vi "Anna_linescan2.0.vi"() -> ()   [LabVIEW 2009]
panel:
  in  "stop batch":bool
  in  "first scan?":bool
  in  "Batch Analyze":bool
  in  "Case Constant\n(See Context Help)":bool
  in  "Router":u32
  in  "save image to txt file":bool
  in  "threshold":cluster{"max":u32, "min":u32}={"max"=100, "min"=20}
  in  "Header Path Ring":u16(ring)
  out "spots":i16
  in  "notes":string="file: 5\r\n13.07.2011 11:31:22\r\n\r\n83 spot(s) found\r\nclose filter:  TRUE\r\nconnectivity 4/8: TRUE\r\nthreshold (min):  20\r\nthreshold (max):  200\r\nselection values:\r\n\r\nNo spots stored.\r\n83 spot(s) found\r\nclose filter:  TRUE\r\nconnectivity 4/8: TRUE\r\nthreshold (min):  20\r\nthreshold (max):  200\r\nselection values:\r\n\r\nNo spots stored.\r\n\r\n\r\nfile: 5\r\n15.07.2011 16:28:43\r\n"
  in  "new image":bool
  in  "exit":bool
  out "does a coinc image exist?":bool
  in  "coincidence spot":bool
  in  "coincidence\nimage":bool
  out "LOADED HDR":bool=TRUE
  out "Image LOADED":bool=TRUE
  in  "settings":bool
  in  "Load Image":bool
  in  "F2-Image":bool
  in  "Lifetime pick":bool
  in  "Export":bool
  in  "TAC Window":bool
  in  "Spotfinder":bool
  in  "View FIFO Settings":bool
  in  "View Image Settings":bool
  in  "Load":bool
  out "total":i32=502376
  out "gap":i32
  out "invalid":i32=69
  in  "plane":u32
  in  "router":u8(ring) items=["sum", "0", "1", "2", "3", "4", "5"]
  in  "RGB or false color?":bool
  in  "16bit":bool
  out "already x spots":i16
  out "Int duplex?":bool
  out "16btimage?":bool
  out "Ampel":cluster{"RED":bool, "YELLOW":bool, "GREEN":bool}={"RED"=FALSE, "YELLOW"=FALSE, "GREEN"=TRUE}
  out "TACwinLoaded?":bool=TRUE
  out "Boolean":bool=TRUE
  in  "Image Path":path=path "C:/Users/Phil/Desktop/11_07_08 Guillermo correlations/silver 40 nm/5/5.hdr"
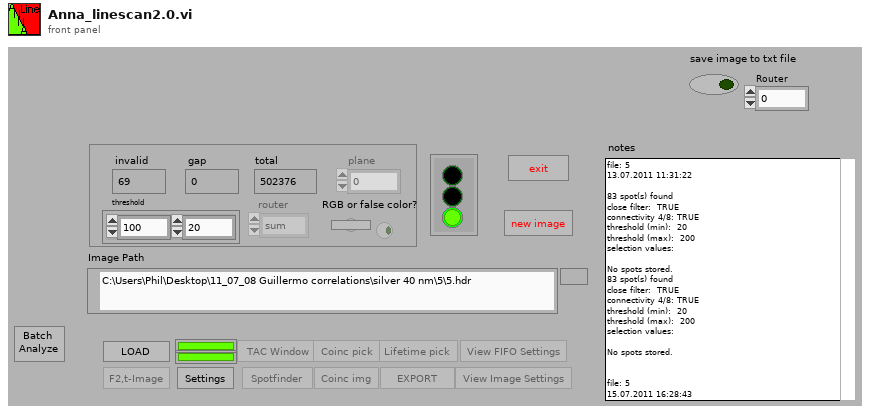
[diagram p1: front panel]
types:
  T1 = enum16{"Display", "change", "get", "save", "create text", "load", "Get Refnum"}
  T2 = enum16{"Get", "Set", "Change", "ini", "clear", "draw", "draw false"}
  T3 = enum16{"Ini", "Get", "Set", "Refresh", "dump", "move", "name"}
  T4 = enum16{"Ini", "Dump", "Colorpal", "Input", "Get"}
  T5 = enum16{"Display", "change", "Get", "Set", "Set Ken"}
  T6 = enum8{"Enabled", "Disabled", "Disabled and Grayed Out"}
  T7 = enum16{"Ini", "Get", "Set", "Draw", "Colorpal", "Dump", "Zoom"}
  T8 = cluster{"router":u8[], "macro times":dbl[], "micro times":u16[], "invalid":dbl[], "gap":dbl[]}
  T9 = typedef "Settings.ctl" = cluster{"threshold":cluster{"max":u32, "min":u32}, "RGB or false color":bool, "16bit":bool, "log/lin axis":u16, "spotsize button":bool, "Pixelsize":u16, "autoscale x":bool, "autoscale y":bool, "correlation":bool, "ADC-Resolution":i32, "F2-lifetime":cluster{"display tau":bool, "display F2":bool, "Palette Number lifetime":enum32{"Gray", "Binary", "Gradient", "Rainbow", "Temperature"}, "Palette Number F2":enum32{"Gray", "Binary", "Gradient", "Rainbow", "Temperature"}, "max tau-Value":dbl, "min tau-Value":dbl, "max F2-Value":dbl, "min F2-Value":dbl}, "TAC-Window 1":u16, "TAC-Window 2":u16, "false color palette":cluster{"1":u32, "2":u32, "3":u32, "4":u32, "5":u32, "6":u32, "7":u32, "8":u32, "8 2":u32, "8 3":u32, "8 4":u32, "8 5":u32}, "rebinning":dbl}
  T10 = enum32{"existing file", "new file", "new or existing file", "existing dir", "new dir", "new or existing dir", "existing file (use LLBs)", "new file (use LLBs)", "new or existing file (use LLBs)", "new or existing file or directory (use LLBs)"}
  T11 = typedef "ImageSettings.ctt" = cluster{"Start Position (µm)":cluster{"x":dbl, "y":dbl, "z":dbl}, "End Position (µm)":cluster{"x":dbl, "y":dbl, "z":dbl}, "Image Resolution (nm/pixel)":cluster{"x":dbl, "y":dbl, "z":dbl}, "Image Size (µm)":cluster{"x":dbl, "y":dbl, "z":dbl}, "Image Size (pixel)":cluster{"x":u32, "y":u32, "z":u32}, "Time Resolution\n(ms/pixel)":dbl, "1st Axis":u16, "2nd Axis":u16, "Retrace":bool, "Estimated Time":string}
  T12 = typedef "FIFOSettings_BH.ctt" = cluster{"Measurement":cluster{"Binning (ms)":sgl, "External Trigger Condition":u16, "Stop Condition:":u16, "Stop Count":dbl, "Buffer Size (Photons)":u16, "No of Channels":u16, "Ext Latch Delay":i16}, "ADC":cluster{"Module":u16, "ADC Resolution":i32, "Dither Range":i16, "Count Increment":i16, "Macro Time Clock":i16}, "SYNC":cluster{"SYNC ZC Level (mV)":sgl, "SYNC Freq Divider":i16, "SYNC Holdoff (ns)":sgl, "SYNC Threshold (mV)":sgl}, "TAC":cluster{"TAC Range (ns)":sgl, "TAC Gain":i16, "TAC Offset (%)":sgl, "TAC Limit Low (%)":sgl, "TAC Limit High (%)":sgl}, "CFD":cluster{"CFD Limit Low (mV)":sgl, "CFD Limit High (mV)":sgl, "CFD ZC Level (mV)":sgl, "CFD Holdoff (ns)":sgl}}
  T13 = typedef "spotproperties.ctl" = cluster{"draw?":bool, "plane":u32, "Coordinates":i32[], "TACWindow":cluster{"TACWindow1":i32, "TACWindow2":i32}, "Lifetime[ns]":ext[], "tauerror":dbl[], "F2-Value overall":dbl, "overall intensity":u32[], "F2-Value TAC":dbl, "TAC intensity":u32[], "Decay":u32[][]}
  T14 = enum16{"open", "replace", "create", "open or create", "replace or create", "replace or create with confirmation"}
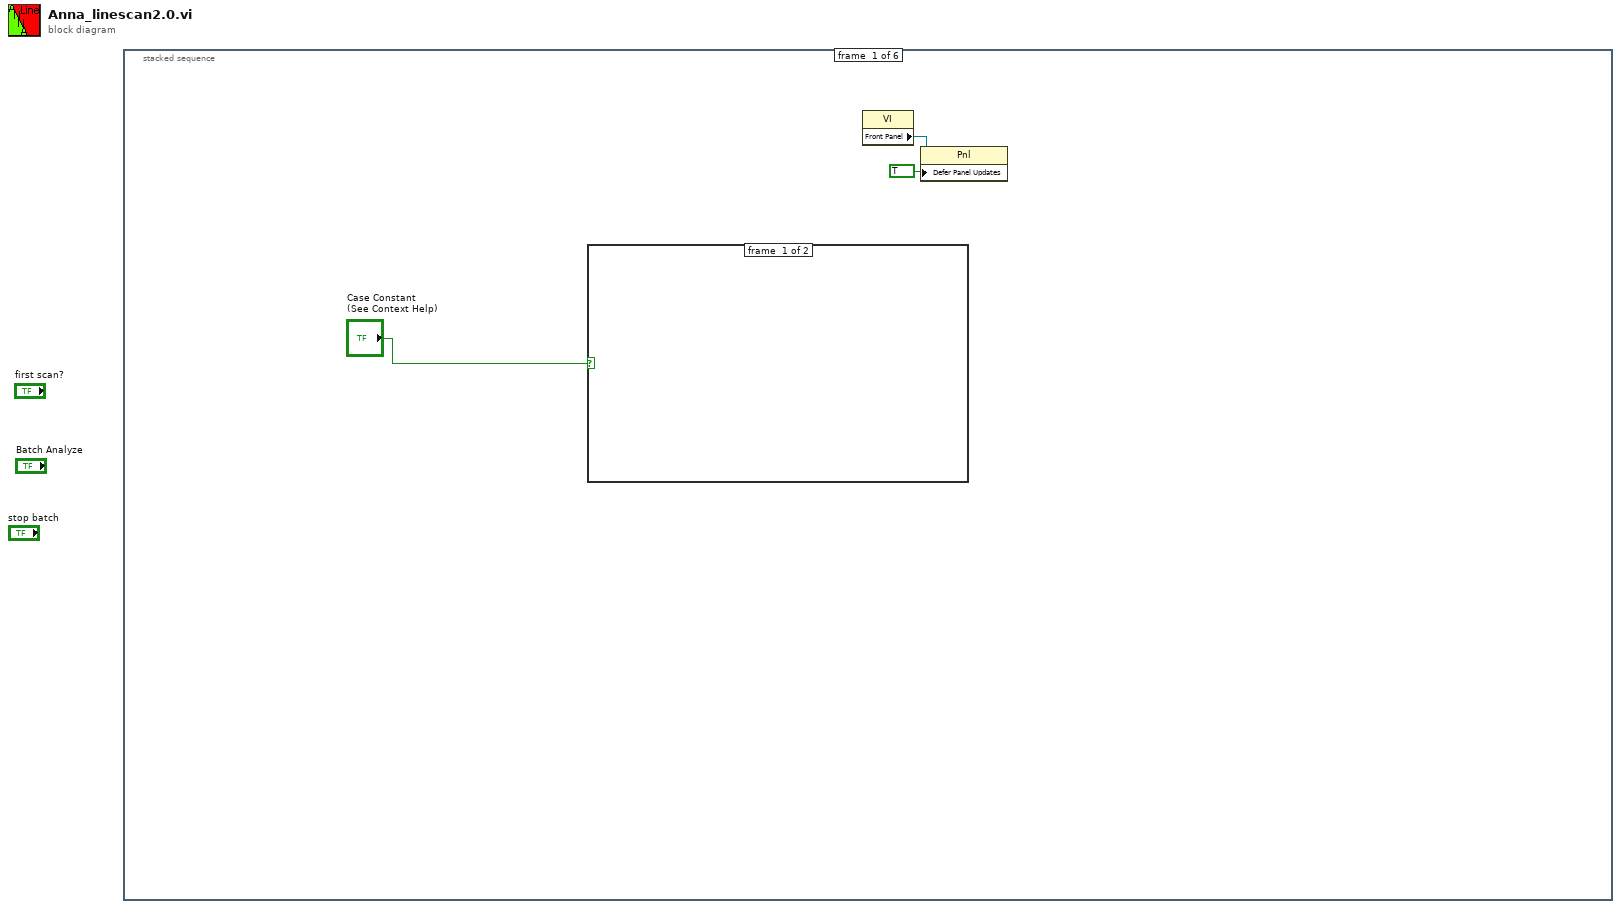
[diagram p0: block diagram]
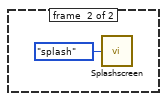
[diagram p2: hidden frame]
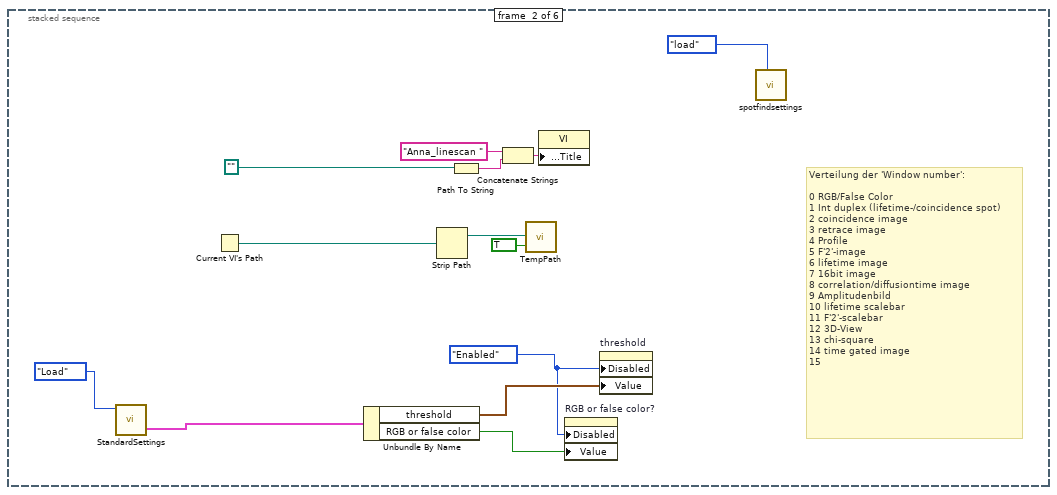
[diagram p3: hidden frame]
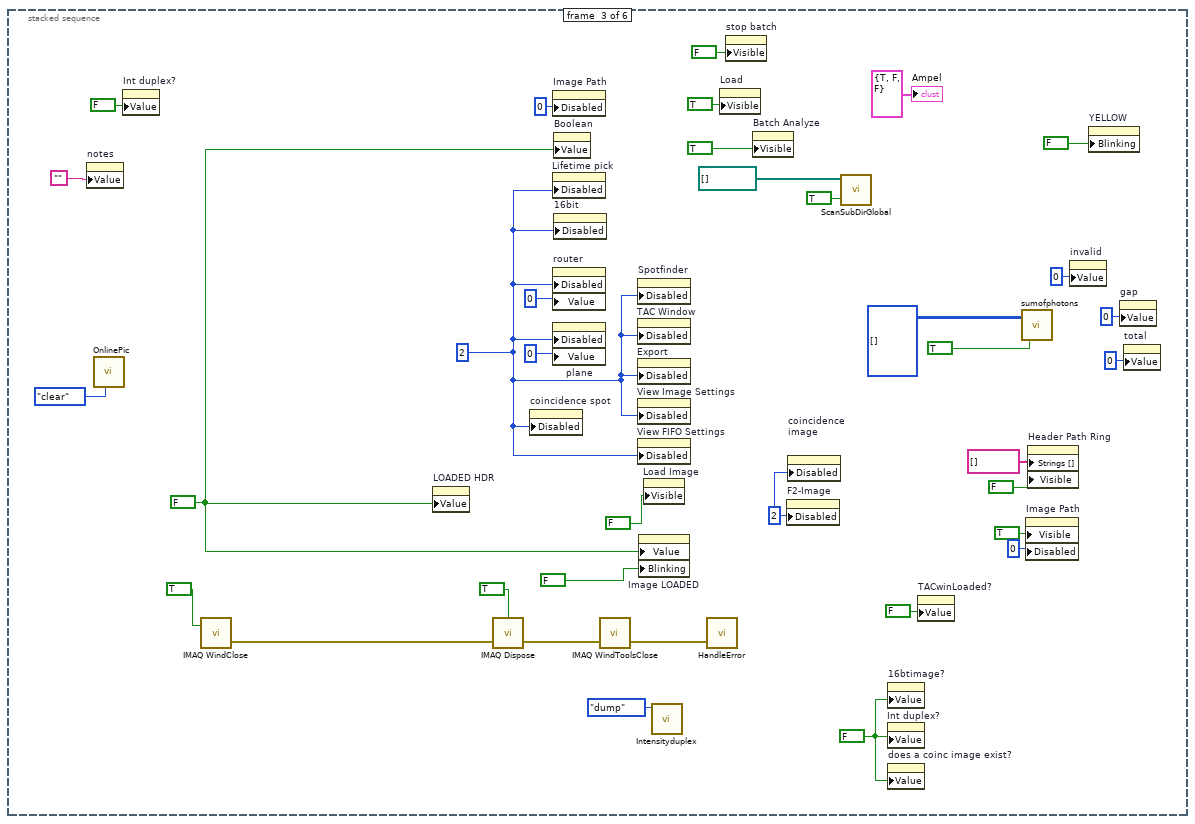
[diagram p4: hidden frame]
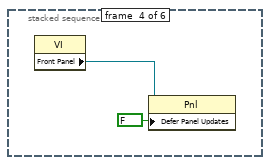
[diagram p5: hidden frame]
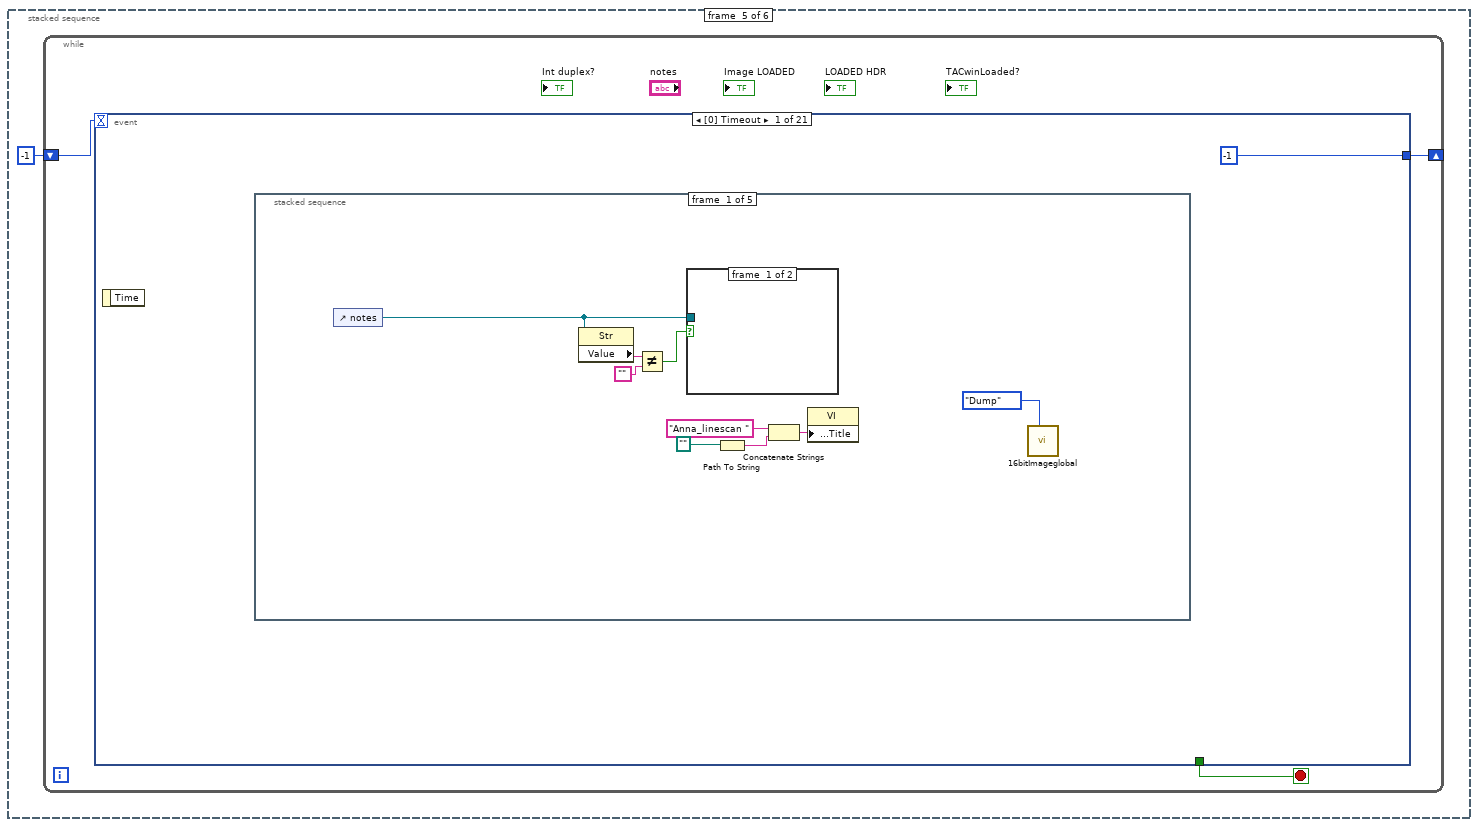
[diagram p6: hidden frame]
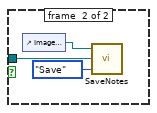
[diagram p7: hidden frame]
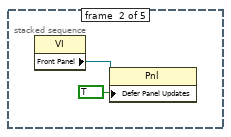
[diagram p8: hidden frame]
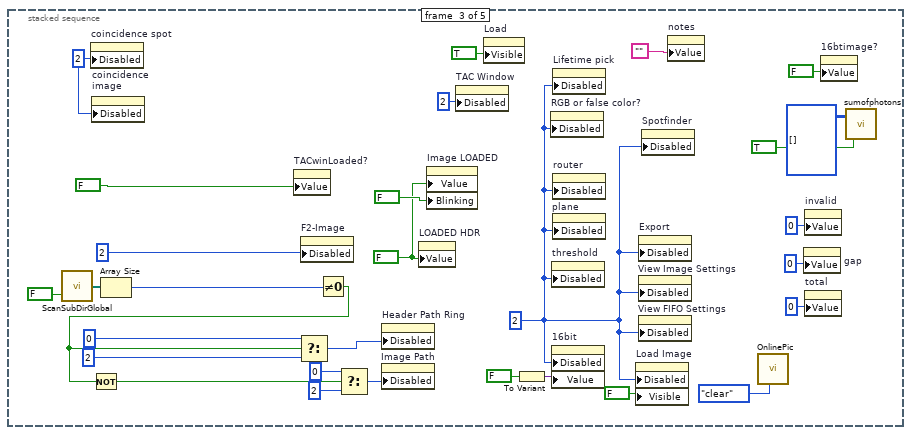
[diagram p9: hidden frame]
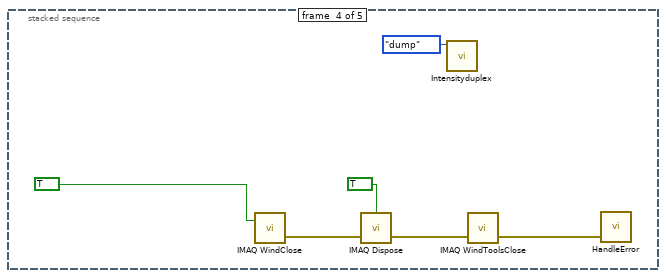
[diagram p10: hidden frame]
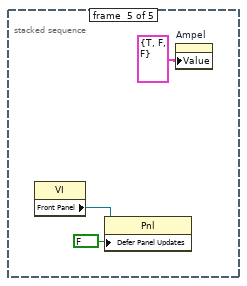
[diagram p11: hidden frame]
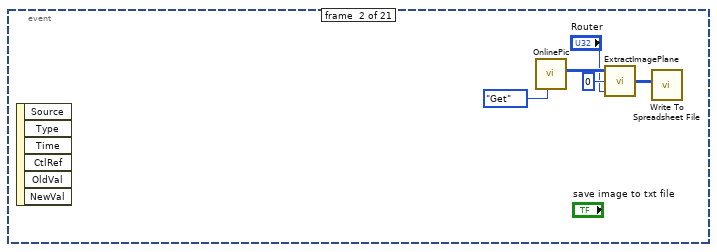
[diagram p12: hidden frame]
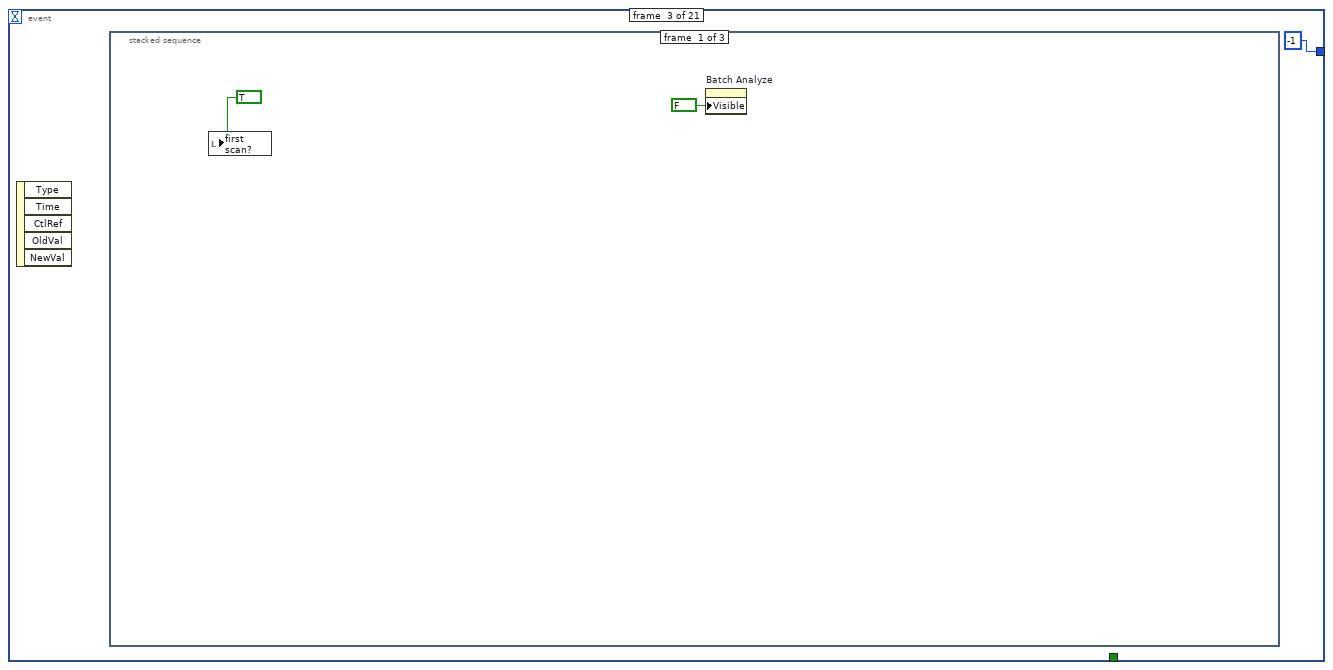
[diagram p13: hidden frame]
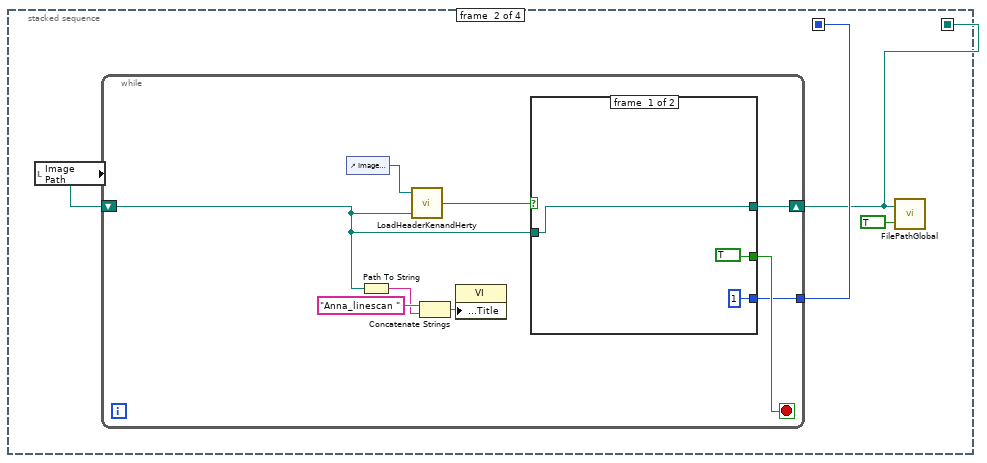
[diagram p15: hidden frame]
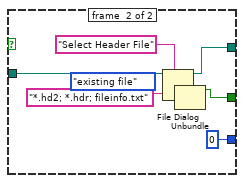
[diagram p16: hidden frame]
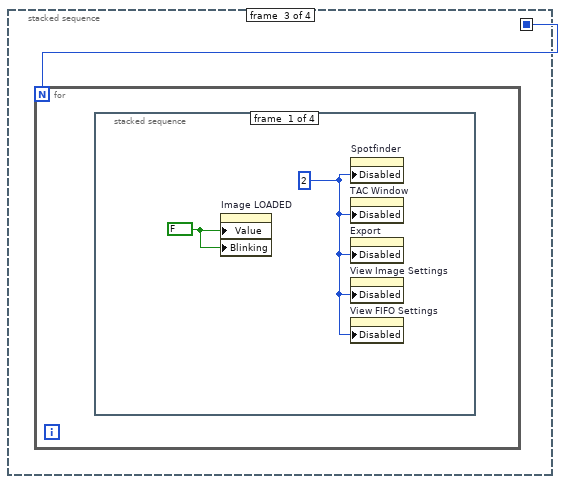
[diagram p17: hidden frame]
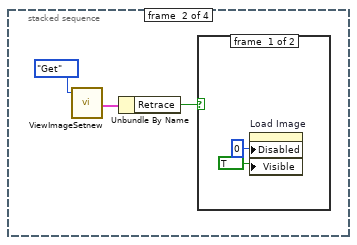
[diagram p18: hidden frame]
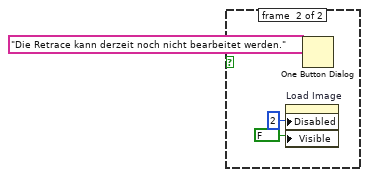
[diagram p19: hidden frame]
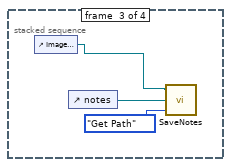
[diagram p20: hidden frame]
diagram:
  n1 = stacked-sequence {
    frame #0 {
      n2 = case shown="False" "Case Constant\n(See Context Help)" {
        frame #0 {
        }
        frame #1 {
          n3 = call "Splashscreen.vi"("Mode"=enum16{"splash", "dialog"}."splash") -> ()  [unwired: 1 in]
        }
      }
      n4 = property class="VI"() -> ("Front Panel"=w2:refnum<vi>)  [unwired: 2 in, 2 out]
      n5 = property class="Pnl"(reference=w2, "Defer Panel Updates"=TRUE) -> ()  [unwired: 1 in, 2 out]
    }
    frame #1 {
      w5 = T6."Enabled" ("Disabled")
      # "Verteilung der 'Window number':\n\n0 RGB/False Color\n1 Int duplex (lifetime-/coincidence spot)\n2 coincidence image\n3 retrace image\n4 Profile\n5 F'2'-image\n6 lifetime image\n7 16bit image\n8 correlation/diffusiontime image\n9 Amplitudenbild\n10 lifetime scalebar\n11 F'2'-scalebar\n12 3D-View\n13 chi-square\n14 time gated image\n15"
      n6 = call "StandardSettings.vi"("Enum"=enum16{"Load", "get", "Save", "set"}."Load") -> ("StandardSettings"=w7:T9)  [unwired: 4 in]
      n7 = Current VI's Path() -> (path=w17:path)
      n8 = Unbundle By Name(w7) -> ("threshold"=w6:cluster{"max":u32, "min":u32}, "RGB or false color"=w8:bool)
      n9 = Strip Path(path=w17) -> (stripped path=w16:path)  [unwired: 1 out]
      n10 = Path To String(path=path "") -> (string=w12:string)
      n11 = Concatenate Strings("Anna_linescan " ("string"), w12) -> (w14:string)
      n12 = call "TempPath.vi"("change"=TRUE, "stripped path"=w16) -> ()  [unwired: 1 in, 1 out]
      n13 = property class="VI"("Front Panel Window:Title"=w14) -> ()  [unwired: 2 in, 2 out]
      n14 = property on="RGB or false color?" class="Boolean (strict)"("Disabled"=w5, "Value"=w8) -> ()  [unwired: 2 in, 2 out]
      n15 = property on="threshold" class="Clust (strict)"("Disabled"=w5, "Value"=w6) -> ()  [unwired: 2 in, 2 out]
      n16 = call "spotfindsettings.vi"("Enum"=T1."load") -> ()  [unwired: 8 in, 3 out]
    }
    frame #2 {
      w33 = FALSE
      w32 = u8 2 ("Disabled")
      w44 = FALSE ("Boolean")
      w22 = u8 2 ("Disabled")
      n17 = property on="notes" class="String"("Value"="") -> ()  [unwired: 2 in, 2 out]
      n18 = call "OnlinePic.vi"("action"=T2."clear" ("Enum")) -> ()  [unwired: 6 in, 5 out]
      n19 = property on="Int duplex?" class="Boolean (strict)"("Value"=FALSE ("Boolean 2")) -> ()  [unwired: 2 in, 2 out]
      n20 = call "IMAQ WindClose"("Close All Windows (False)"=TRUE ("Close All Windows (N)")) -> ("error out"=w49:errorcluster)  [unwired: 5 in]
      n21 = property on="LOADED HDR" class="Bool (strict)"("Value"=w44) -> ()  [unwired: 2 in, 2 out]
      n22 = call "IMAQ Dispose"("All Images? (No)"=TRUE, "error in (no error)"=w49) -> ("error out"=w50:errorcluster)  [unwired: 4 in]
      n23 = property on="coincidence spot" class="Boolean"("Disabled"=w22) -> ()  [unwired: 2 in, 2 out]
      n24 = property on="Image Path" class="Path"("Disabled"=u8 0) -> ()  [unwired: 2 in, 2 out]
      n25 = property on="Lifetime pick" class="Boolean"("Disabled"=w22) -> ()  [unwired: 2 in, 2 out]
      n26 = property on="router" class="Ring (strict)"("Disabled"=w22, "Value"=u8 0 ("router")) -> ()  [unwired: 2 in, 2 out]
      n27 = property on="plane" class="DigNum (strict)"("Disabled"=w22, "Value"=u32 0 ("plane")) -> ()  [unwired: 2 in, 2 out]
      n28 = property on="Boolean" class="Bool (strict)"("Value"=w44) -> ()  [unwired: 2 in, 2 out]
      n29 = property on="16bit" class="Boolean"("Disabled"=w22) -> ()  [unwired: 2 in, 2 out]
      n30 = call "IMAQ WindToolsClose"("error in (no error)"=w50) -> ("error out"=w48:errorcluster)  [unwired: 5 in]
      n31 = property on="Spotfinder" class="Boolean"("Disabled"=w22) -> ()  [unwired: 2 in, 2 out]
      n32 = property on="TAC Window" class="Boolean"("Disabled"=w22) -> ()  [unwired: 2 in, 2 out]
      n33 = property on="Export" class="Boolean"("Disabled"=w22) -> ()  [unwired: 2 in, 2 out]
      n34 = property on="View Image Settings" class="Boolean"("Disabled"=w22) -> ()  [unwired: 2 in, 2 out]
      n35 = property on="View FIFO Settings" class="Boolean"("Disabled"=w22) -> ()  [unwired: 2 in, 2 out]
      n36 = property on="Image LOADED" class="Boolean (strict)"("Value"=w44, "Blinking"=FALSE) -> ()  [unwired: 2 in, 2 out]
      n37 = property on="Load Image" class="Boolean"("Visible"=FALSE) -> ()  [unwired: 2 in, 2 out]
      n38 = call "Intensityduplex.vi"("Enum"=T3."dump") -> ()  [unwired: 4 in, 2 out]
      n39 = call "HandleError.vi"("error in (no error)"=w48) -> ()
      n40 = property on="Load" class="Bool"("Visible"=TRUE) -> ()  [unwired: 2 in, 2 out]
      n41 = property on="stop batch" class="Bool (strict)"("Visible"=FALSE) -> ()  [unwired: 2 in, 2 out]
      n42 = property on="Batch Analyze" class="Bool"("Visible"=TRUE) -> ()  [unwired: 2 in, 2 out]
      n43 = property on="F2-Image" class="Boolean"("Disabled"=w32) -> ()  [unwired: 2 in, 2 out]
      n44 = property on="coincidence\nimage" class="Bool"("Disabled"=w32) -> ()  [unwired: 2 in, 2 out]
      n45 = call "ScanSubDirGlobal.vi"("set"=TRUE, "Array 2"=path[] []) -> ()  [unwired: 1 out]
      n46 = property on="16btimage?" class="Boolean (strict)"("Value"=w33) -> ()  [unwired: 2 in, 2 out]
      n47 = property on="Int duplex?" class="Boolean (strict)"("Value"=w33) -> ()  [unwired: 2 in, 2 out]
      n48 = property on="does a coinc image exist?" class="Boolean (strict)"("Value"=w33) -> ()  [unwired: 2 in, 2 out]
      n49 = property on="TACwinLoaded?" class="Boolean (strict)"("Value"=FALSE ("TACwinLoaded?")) -> ()  [unwired: 2 in, 2 out]
      n50 = call "sumofphotons.vi"("s"=TRUE, "sum of photons"=u32[][][][] []) -> ()  [unwired: 1 out]
      n51 = property on="Image Path" class="Path"("Visible"=TRUE, "Disabled"=u8 0) -> ()  [unwired: 2 in, 2 out]
      n52 = property on="Header Path Ring" class="Ring (strict)"("Strings []"=string[] [], "Visible"=FALSE) -> ()  [unwired: 2 in, 2 out]
      n53 = property on="invalid" class="DigNum (strict)"("Value"=u32 0 ("invalid photons")) -> ()  [unwired: 2 in, 2 out]
      n54 = property on="YELLOW" class="Boolean (strict)"("Blinking"=FALSE) -> ()  [unwired: 2 in, 2 out]
      n55 = property on="gap" class="DigNum (strict)"("Value"=u32 0 ("gap photons")) -> ()  [unwired: 2 in, 2 out]
      n56 = property on="total" class="DigNum (strict)"("Value"=u32 0 ("invalid photons")) -> ()  [unwired: 2 in, 2 out]
      "Ampel" <- cluster{"RED":bool, "YELLOW":bool, "GREEN":bool} {"RED"=TRUE, "YELLOW"=FALSE, "GREEN"=FALSE} ("Ampel")
    }
    frame #3 {
      n57 = property class="VI"() -> ("Front Panel"=w53:refnum<vi>)  [unwired: 2 in, 2 out]
      n58 = property class="Pnl"(reference=w53, "Defer Panel Updates"=FALSE) -> ()  [unwired: 1 in, 2 out]
    }
    frame #4 {
      n59 = while {
        shift-right: [w57] -> _
        shift-left: -1 -> [w56]
        stop <- w58 stop-if-true
        n60 = event shown="[0] Timeout" {
          selector: _ -> [_ _ _ _ _ _ _ _ _ _ _ _ _ _ _ _ _ _ _ _ _]
          dyn-events: _ -> [_ _ _ _ _ _ _ _ _ _ _ _ _ _ _ _ _ _ _ _ _]
          timeout: w56 -> [_ _ _ _ _ _ _ _ _ _ _ _ _ _ _ _ _ _ _ _ _]
          tunnel: [_ _ _ _ _ _ FALSE ("T button?") _ _ _ _ _ _ _ _ _ _ w612 _ TRUE w991] -> w58
          tunnel: [-1 _ -1 -1 -1 -1 -1 100 -1 -1 -1 -1 -1 -1 -1 -1 -1 -1 -1 _ _] -> w57
          event #0 {
            n61 = event-data() -> ()  [unwired: 1 in, 1 out]
            n62 = stacked-sequence {
              frame #0 {
                n63 = control-ref of="notes"() -> (w68:refnum<vi>)
                n64 = property class="Str"(reference=w68) -> ("Value"=w61:string)  [unwired: 1 in, 2 out]
                n65 = Not Equal?(x=w61, y="") -> (x != y?=w60:bool)
                n66 = case shown="True" w60 {
                  tunnel: w68 -> [_ w70]
                  frame #0 {
                  }
                  frame #1 {
                    n67 = control-ref of="Image Path"() -> (w69:refnum<vi>)
                    n68 = call "SaveNotes.vi"("Enum"=enum16{"Get Path", "Read", "Save"}."Save", "String"=w70, "Path"=w69) -> ()  [unwired: 2 in]
                  }
                }
                n69 = Path To String(path=path "") -> (string=w65:string)
                n70 = Concatenate Strings("Anna_linescan " ("string"), w65) -> (w67:string)
                n71 = property class="VI"("Front Panel Window:Title"=w67) -> ()  [unwired: 2 in, 2 out]
                n72 = call "16bitImageglobal.vi"("Enum"=T4."Dump") -> ()  [unwired: 4 in, 4 out]
              }
              frame #1 {
                n73 = property class="VI"() -> ("Front Panel"=w72:refnum<vi>)  [unwired: 2 in, 2 out]
                n74 = property class="Pnl"(reference=w72, "Defer Panel Updates"=TRUE) -> ()  [unwired: 1 in, 2 out]
              }
              frame #2 {
                w83 = u8 2 ("Disabled")
                w79 = FALSE ("Boolean")
                w74 = u8 2 ("Disabled")
                n75 = call "ScanSubDirGlobal.vi"("set"=FALSE) -> ("Array"=w92:path[])  [unwired: 1 in]
                n76 = property on="coincidence spot" class="Bool"("Disabled"=w83) -> ()  [unwired: 2 in, 2 out]
                n77 = property on="coincidence\nimage" class="Bool"("Disabled"=w83) -> ()  [unwired: 2 in, 2 out]
                n78 = Array Size(array=w92) -> (size(s)=w91:i32)
                n79 = property on="TACwinLoaded?" class="Boolean (strict)"("Value"=FALSE ("TACwinLoaded?")) -> ()  [unwired: 2 in, 2 out]
                n80 = property on="F2-Image" class="Boolean"("Disabled"=u8 2) -> ()  [unwired: 2 in, 2 out]
                n81 = Not Equal To 0?(x=w91) -> (x != 0?=w88:bool)
                n82 = Not(x=w88) -> (.not. x?=w87:bool)
                n83 = Select(t=u8 0 ("Disabled"), s=w88, f=u8 2 ("Disabled")) -> (s? t:f=w86:u8)
                n84 = Select(t=u8 0 ("Disabled"), s=w87, f=u8 2 ("Disabled")) -> (s? t:f=w85:u8)
                n85 = property on="Header Path Ring" class="Ring (strict)"("Disabled"=w86) -> ()  [unwired: 2 in, 2 out]
                n86 = property on="Image Path" class="Path"("Disabled"=w85) -> ()  [unwired: 2 in, 2 out]
                n87 = property on="LOADED HDR" class="Bool (strict)"("Value"=w79) -> ()  [unwired: 2 in, 2 out]
                n88 = property on="Image LOADED" class="Boolean (strict)"("Value"=w79, "Blinking"=FALSE) -> ()  [unwired: 2 in, 2 out]
                n89 = property on="TAC Window" class="Boolean"("Disabled"=2) -> ()  [unwired: 2 in, 2 out]
                n90 = property on="Load" class="Bool"("Visible"=TRUE) -> ()  [unwired: 2 in, 2 out]
                n91 = To Variant(anything=FALSE ("16btimage?")) -> (Variant=w76:variant)
                n92 = property on="RGB or false color?" class="Boolean (strict)"("Disabled"=w74) -> ()  [unwired: 2 in, 2 out]
                n93 = property on="threshold" class="Clust (strict)"("Disabled"=w74) -> ()  [unwired: 2 in, 2 out]
                n94 = property on="16bit" class="Boolean"("Disabled"=w74, "Value"=w76) -> ()  [unwired: 2 in, 2 out]
                n95 = property on="Lifetime pick" class="Boolean"("Disabled"=w74) -> ()  [unwired: 2 in, 2 out]
                n96 = property on="router" class="Ring (strict)"("Disabled"=w74) -> ()  [unwired: 2 in, 2 out]
                n97 = property on="plane" class="DigNum (strict)"("Disabled"=w74) -> ()  [unwired: 2 in, 2 out]
                n98 = property on="Load Image" class="Boolean"("Disabled"=w74, "Visible"=FALSE) -> ()  [unwired: 2 in, 2 out]
                n99 = property on="Export" class="Boolean"("Disabled"=w74) -> ()  [unwired: 2 in, 2 out]
                n100 = property on="View Image Settings" class="Boolean"("Disabled"=w74) -> ()  [unwired: 2 in, 2 out]
                n101 = property on="View FIFO Settings" class="Boolean"("Disabled"=w74) -> ()  [unwired: 2 in, 2 out]
                n102 = property on="Spotfinder" class="Boolean"("Disabled"=w74) -> ()  [unwired: 2 in, 2 out]
                n103 = property on="notes" class="String"("Value"="") -> ()  [unwired: 2 in, 2 out]
                n104 = call "OnlinePic.vi"("action"=T2."clear" ("Enum")) -> ()  [unwired: 6 in, 5 out]
                n105 = property on="gap" class="DigNum (strict)"("Value"=u32 0 ("gap photons")) -> ()  [unwired: 2 in, 2 out]
                n106 = property on="invalid" class="DigNum (strict)"("Value"=u32 0 ("invalid photons")) -> ()  [unwired: 2 in, 2 out]
                n107 = property on="total" class="DigNum (strict)"("Value"=u32 0 ("invalid photons")) -> ()  [unwired: 2 in, 2 out]
                n108 = property on="16btimage?" class="Boolean (strict)"("Value"=FALSE ("16btimage?")) -> ()  [unwired: 2 in, 2 out]
                n109 = call "sumofphotons.vi"("s"=TRUE, "sum of photons"=u32[][][][] []) -> ()  [unwired: 1 out]
              }
              frame #3 {
                n110 = call "IMAQ WindClose"("Close All Windows (False)"=TRUE ("Close All Windows (N)")) -> ("error out"=w107:errorcluster)  [unwired: 5 in]
                n111 = call "IMAQ Dispose"("All Images? (No)"=TRUE, "error in (no error)"=w107) -> ("error out"=w108:errorcluster)  [unwired: 4 in]
                n112 = call "Intensityduplex.vi"("Enum"=T3."dump") -> ()  [unwired: 4 in, 2 out]
                n113 = call "IMAQ WindToolsClose"("error in (no error)"=w108) -> ("error out"=w104:errorcluster)  [unwired: 5 in]
                n114 = call "HandleError.vi"("error in (no error)"=w104) -> ()
              }
              frame #4 {
                n115 = property class="VI"() -> ("Front Panel"=w110:refnum<vi>)  [unwired: 2 in, 2 out]
                n116 = property class="Pnl"(reference=w110, "Defer Panel Updates"=FALSE) -> ()  [unwired: 1 in, 2 out]
                n117 = property on="Ampel" class="Clust (strict)"("Value"=cluster{"RED":bool, "RED 2":bool, "RED 3":bool} {"RED"=TRUE, "RED 2"=FALSE, "RED 3"=FALSE} ("Ampel")) -> ()  [unwired: 2 in, 2 out]
              }
            }
          }
          event #1 {
            n118 = event-data() -> ()  [unwired: 1 in, 6 out]
            n119 = call "OnlinePic.vi"("action"=enum16{"Get", "Set", "Change", "ini"}."Get" ("Enum")) -> ("Sum of Photons"=w116:u32[][][][])  [unwired: 6 in, 4 out]
            n120 = call "ExtractImagePlane.vi"("Router"="Router", "Plane"=u32 0, "Trace"=w116) -> ("Intensity"=w113:u32[][])
            n121 = call "Write To Spreadsheet File.vi"("2D data"=w113) -> ()  [unwired: 7 in, 1 out]
          }
          event #2 {
            n122 = event-data() -> ()  [unwired: 1 in, 5 out]
            n123 = stacked-sequence {
              frame #0 {
                n124 = local write "first scan?"(TRUE ("first scan?")) -> ()
                n125 = property on="Batch Analyze" class="Bool"("Visible"=FALSE) -> ()  [unwired: 2 in, 2 out]
              }
              frame #1 {
                n126 = while {
                  stop <- w121 continue-if-true
                  n127 = stacked-sequence {
                    seq-local: [_ w125 _ _] -> [_ _ w145 _]
                    seq-local: [_ w122 _ _] -> [_ _ _ w163]
                    tunnel: [_ _ _ w162] -> w121
                    frame #0 {
                    }
                    frame #1 {
                      n128 = local read "Image Path"() -> (w123:path)
                      n129 = while {
                        shift-right: [w127] -> w122
                        shift-left: w123 -> [w128]
                        tunnel: [w126] -> w125
                        stop <- w129 stop-if-true
                        n130 = control-ref of="Image Path"() -> (w134:refnum<vi>)
                        n131 = Path To String(path=w128) -> (string=w131:string)
                        n132 = call "LoadHeaderKenandHerty.vi"("appended path"=w128, "reference"=w134) -> ("unsuccesful?"=w130:bool)  [unwired: 3 in]
                        n133 = Concatenate Strings("Anna_linescan " ("string"), w131) -> (w133:string)
                        n134 = property class="VI"("Front Panel Window:Title"=w133) -> ()  [unwired: 2 in, 2 out]
                        n135 = case shown="False" w130 {
                          tunnel: w128 -> [w135 w144]
                          tunnel: [TRUE w140] -> w129
                          tunnel: [w135 w142] -> w127
                          tunnel: [1 0] -> w126
                          frame #0 {
                          }
                          frame #1 {
                            (unwired) T10."existing file" ("select mode (2)")
                            n136 = File Dialog(6:"*.hd2; *.hdr; fileinfo.txt" ("pattern"), 7:"Select Header File" ("prompt"), 11:w144) -> (0:w138:errorcluster, 1:w140:bool, 3:w142:path)  [unwired: 4 in, 1 out]
                            n137 = Unbundle(w138) -> ()  [unwired: 3 out]
                          }
                        }
                      }
                      n138 = call "FilePathGlobal.vi"("Image Path"=w122, "set?"=TRUE) -> ()  [unwired: 3 out]
                    }
                    frame #2 {
                      n139 = for {
                        N: w145 -> [_]
                        n140 = stacked-sequence {
                          frame #0 {
                            w147 = u8 2 ("Disabled")
                            w146 = FALSE ("Boolean")
                            n141 = property on="Image LOADED" class="Boolean (strict)"("Value"=w146, "Blinking"=w146) -> ()  [unwired: 2 in, 2 out]
                            n142 = property on="Spotfinder" class="Boolean"("Disabled"=w147) -> ()  [unwired: 2 in, 2 out]
                            n143 = property on="TAC Window" class="Boolean"("Disabled"=w147) -> ()  [unwired: 2 in, 2 out]
                            n144 = property on="Export" class="Boolean"("Disabled"=w147) -> ()  [unwired: 2 in, 2 out]
                            n145 = property on="View Image Settings" class="Boolean"("Disabled"=w147) -> ()  [unwired: 2 in, 2 out]
                            n146 = property on="View FIFO Settings" class="Boolean"("Disabled"=w147) -> ()  [unwired: 2 in, 2 out]
                          }
                          frame #1 {
                            n147 = call "ViewImageSetnew.vi"("action"=enum16{"Display", "change", "Get", "Set"}."Get" ("Enum")) -> ("Image Settings"=w149:T11)  [unwired: 2 in]
                            n148 = Unbundle By Name(w149) -> ("Retrace"=w148:bool)
                            n149 = case shown="False" w148 {
                              frame #0 {
                                n150 = property on="Load Image" class="Boolean"("Disabled"=u8 0, "Visible"=TRUE) -> ()  [unwired: 2 in, 2 out]
                              }
                              frame #1 {
                                n151 = property on="Load Image" class="Boolean"("Disabled"=u8 2, "Visible"=FALSE) -> ()  [unwired: 2 in, 2 out]
                                n152 = One Button Dialog(message="Die Retrace kann derzeit noch nicht bearbeitet werden.") -> ()  [unwired: 1 in, 1 out]
                              }
                            }
                          }
                          frame #2 {
                            n153 = control-ref of="Image Path"() -> (w156:refnum<vi>)
                            n154 = control-ref of="notes"() -> (w158:refnum<vi>)
                            n155 = call "SaveNotes.vi"("Enum"=enum16{"Get Path", "Read", "Save"}."Get Path", "String"=w158, "Path"=w156) -> ()  [unwired: 2 in]
                          }
                          frame #3 {
                            (unwired) FALSE ("Visible")
                            w160 = u8 0 ("Disabled")
                            n156 = property on="Image LOADED" class="Boolean (strict)"("Disabled"=w160) -> ()  [unwired: 2 in, 2 out]
                            n157 = property on="View Image Settings" class="Boolean"("Disabled"=w160) -> ()  [unwired: 2 in, 2 out]
                            n158 = property on="View FIFO Settings" class="Boolean"("Disabled"=w160) -> ()  [unwired: 2 in, 2 out]
                            n159 = property on="LOADED HDR" class="Bool (strict)"("Value"=TRUE ("Boolean")) -> ()  [unwired: 2 in, 2 out]
                            n160 = property on="Ampel" class="Clust (strict)"("Value"=cluster{"RED":bool, "RED 2":bool, "RED 3":bool} {"RED"=TRUE, "RED 2"=TRUE, "RED 3"=FALSE} ("Ampel")) -> ()  [unwired: 2 in, 2 out]
                          }
                        }
                      }
                    }
                    frame #3 {
                      n161 = stacked-sequence {
                        tunnel: w163 -> [_ _ _ _ _ _ _ _ _ _ _ w260]
                        tunnel: [_ _ _ _ _ _ _ _ _ _ _ w259] -> w162
                        frame #0 {
                          n162 = property on="Image LOADED" class="Bool (strict)"("Blinking"=TRUE) -> ()  [unwired: 2 in, 2 out]
                          n163 = property on="Image Path" class="Path"("Disabled"=u8 2) -> ()  [unwired: 2 in, 2 out]
                          n164 = property on="Load Image" class="Bool"("Disabled"=u8 2) -> ()  [unwired: 2 in, 2 out]
                          n165 = call "sumofphotons.vi"("s"=TRUE, "sum of photons"=u32[][][][] []) -> ()  [unwired: 1 out]
                        }
                        frame #1 {
                          n166 = call "WriteTempData.vi"("Enum"=enum16{"create new", "write", "close"}."create new") -> ("error out"=w169:errorcluster)  [unwired: 4 in, 1 out]
                          n167 = call "HandleError.vi"("error in (no error)"=w169) -> ()
                        }
                        frame #2 {
                          n168 = call "fileformatGlobal.vi"("changed"=FALSE) -> ("fileformat out"=w171:enum16{"Herty", "Ken", "SPC130", "HydraHarp"})  [unwired: 1 in]
                          n169 = control-ref of="Image Path"() -> (w173:refnum<vi>)
                          n170 = case shown="\"Herty\", Default" w171 {
                            tunnel: w173 -> [w174 w175 w176 w177]
                            frame #0 {
                              n171 = call "LoadData.vi"("Path"=w174) -> ()  [unwired: 2 in, 3 out]
                            }
                            frame #1 {
                              n172 = call "LoadDataSPC130.vi"("Path"=w175) -> ()  [unwired: 2 in, 3 out]
                            }
                            frame #2 {
                              n173 = call "LoadDataHH.vi"("Path"=w176) -> ()  [unwired: 2 in, 3 out]
                            }
                            frame #3 {
                              n174 = call "LoadDataKen.vi"("Path"=w177) -> ()  [unwired: 5 in]
                            }
                          }
                        }
                        frame #3 {
                          n175 = call "WriteTempData.vi"("Enum"=enum16{"create new", "write", "close"}."close") -> ("error out"=w178:errorcluster)  [unwired: 4 in, 1 out]
                          n176 = call "HandleError.vi"("error in (no error)"=w178) -> ()
                        }
                        frame #4 {
                          n177 = call "TotalRecall_Reload.vi"() -> ("gap"=w182:i32, "invalid"=w181:i32, "valid"=w180:i32)  [unwired: 4 in, 1 out]
                          n178 = property on="gap" class="DigNum (strict)"("Value"=w182) -> ()  [unwired: 2 in, 2 out]
                          n179 = property on="invalid" class="DigNum (strict)"("Value"=w181) -> ()  [unwired: 2 in, 2 out]
                          n180 = property on="total" class="DigNum (strict)"("Value"=w180) -> ()  [unwired: 2 in, 2 out]
                        }
                        frame #5 {
                          n181 = call "ViewFIFOSet.vi"("Enum"=T5."Get") -> ("FIFO Settings (Array)"=w189:T12[])  [unwired: 1 in]
                          n182 = Index Array(array=w189) -> (element=w190:T12)  [unwired: 1 in]
                          n183 = Array Size(array=w189) -> (size(s)=w185:i32)
                          n184 = Unbundle By Name(w190) -> ("Measurement.No of Channels"=w184:u16)
                          n185 = Multiply(x=w184, y=w185) -> (x*y=w183:i32)
                          n186 = for {
                            N: w183 -> [_]
                            tunnel: [w199] -> w188 mode=indexing
                            i -> [w200]
                            n187 = Number To Decimal String(number=w200) -> (decimal integer string=w199:string)  [unwired: 1 in]
                          }
                          n188 = Build Array (concatenate)("sum", w188) -> (w186:string[])
                          n189 = property on="router" class="Ring (strict)"("Strings []"=w186) -> ("Value"=w195:u8)  [unwired: 2 in, 2 out]
                          n190 = property on="plane" class="DigNum (strict)"() -> ("Value"=w196:u32)  [unwired: 2 in, 2 out]
                          n191 = property on="threshold" class="Clust (strict)"() -> ("Value"=w192:cluster{"max":u32, "min":u32})  [unwired: 2 in, 2 out]
                          n192 = call "sumofphotons.vi"("s"=FALSE) -> ("sum of photons out"=w193:u32[][][][])  [unwired: 1 in]
                          n193 = property on="RGB or false color?" class="Bool (strict)"() -> ("Value"=w197:bool)  [unwired: 2 in, 2 out]
                          n194 = call "OnlinePic.vi"("action"=T2."ini" ("Enum"), "RGB/False"=w197, "Threshold (max)"=w192, "plane"=w196, "router channel"=w195, "Array"=w193) -> ()  [unwired: 1 in, 5 out]
                        }
                        frame #6 {
                          n195 = call "ViewImageSetnew.vi"("action"=enum16{"Display", "change", "Get", "Set"}."Get" ("Enum")) -> ("Image Settings"=w202:T11)  [unwired: 2 in]
                          n196 = Unbundle By Name(w202) -> ("Image Size (pixel).z"=w203:u32)
                          n197 = case shown="0" w203 {
                            tunnel: [i8 2 w208] -> w204
                            tunnel: [u8 0 w208] -> w205
                            frame #0 {
                            }
                            frame #1 {
                              w208 = u8 0
                            }
                          }
                          n198 = property on="plane" class="DigNum (strict)"("Disabled"=w204, "Value"=w205) -> ()  [unwired: 2 in, 2 out]
                        }
                        frame #7 {
                          w209 = u8 0
                          n199 = property on="Image LOADED" class="Bool (strict)"("Blinking"=FALSE, "Value"=TRUE ("Image LOADED")) -> ()  [unwired: 2 in, 2 out]
                          n200 = property on="Lifetime pick" class="Bool"("Disabled"=w209) -> ()  [unwired: 2 in, 2 out]
                          n201 = property on="RGB or false color?" class="Bool (strict)"("Disabled"=w209) -> ()  [unwired: 2 in, 2 out]
                          n202 = property on="16bit" class="Bool"("Disabled"=w209) -> ()  [unwired: 2 in, 2 out]
                          n203 = property on="threshold" class="Clust (strict)"("Disabled"=w209) -> ()  [unwired: 2 in, 2 out]
                          n204 = property on="Spotfinder" class="Bool"("Disabled"=w209) -> ()  [unwired: 2 in, 2 out]
                          n205 = property on="router" class="Ring (strict)"("Disabled"=w209) -> ()  [unwired: 2 in, 2 out]
                          n206 = property on="coincidence spot" class="Bool"("Disabled"=w209) -> ()  [unwired: 2 in, 2 out]
                          n207 = property on="TAC Window" class="Bool"("Disabled"=w209) -> ()  [unwired: 2 in, 2 out]
                          n208 = property on="Export" class="Bool"("Disabled"=w209) -> ()  [unwired: 2 in, 2 out]
                          n209 = property on="F2-Image" class="Bool"("Disabled"=u8 0) -> ()  [unwired: 2 in, 2 out]
                          n210 = property on="coincidence\nimage" class="Bool"("Disabled"=w209) -> ()  [unwired: 2 in, 2 out]
                        }
                        frame #8 {
                          n211 = property on="Ampel" class="Clust (strict)"("Value"=cluster{"RED":bool, "RED 2":bool, "RED 3":bool} {"RED"=FALSE, "RED 2"=FALSE, "RED 3"=TRUE} ("Ampel")) -> ()  [unwired: 2 in, 2 out]
                        }
                        frame #9 {
                          # "settings and TAC Window pop up only for first scan!"
                          n212 = local read "first scan?"() -> (w214:bool)
                          n213 = case shown="True" w214 {
                            frame #0 {
                            }
                            frame #1 {
                              n214 = stacked-sequence {
                                frame #0 {
                                n215 = control-ref of="Image Path"() -> (w215:refnum<vi>)
                                n216 = call "GetSetTempDir.vi"("Path"=w215) -> ()  [unwired: 4 in]
                                }
                                frame #1 {
                                n217 = property on="Ampel" class="Clust (strict)"("Value"=cluster{"RED":bool, "RED 2":bool, "RED 3":bool} {"RED"=FALSE, "RED 2"=FALSE, "RED 3"=FALSE} ("Ampel")) -> ()  [unwired: 2 in, 2 out]
                                n218 = property on="YELLOW" class="Bool (strict)"("Blinking"=TRUE) -> ()  [unwired: 2 in, 2 out]
                                }
                                frame #2 {
                                n219 = property on="Image LOADED" class="Bool (strict)"() -> ("Value"=w218:bool)  [unwired: 2 in, 2 out]
                                n220 = case shown="True" w218 {
                                frame #0 {
                                }
                                frame #1 {
                                n221 = call "GetTACWindow.vi"("Enum"=enum16{"ini", "get", "quick"}."ini") -> ("Cursor.Cursor Position:Cursor X"=w227:u16, "Cursor.Cursor Position:Cursor X 2"=w228:u16, "x-values"=w221:dbl[], "ready?"=w222:bool)  [unwired: 1 in, 5 out]
                                n222 = Select(t=2, s=w222, f=0) -> (s? t:f=w225:i32)
                                n223 = property on="TACwinLoaded?" class="Bool (strict)"("Value"=TRUE ("TACwinLoaded?")) -> ()  [unwired: 2 in, 2 out]
                                n224 = call "CursorPositionChanged.vi"("CursorPos x1"=w228, "CursorPos x0"=w227, "x-values"=w221, "action"=enum16{"Check", "Get", "xval"}."xval" ("Enum")) -> ()  [unwired: 4 out]
                                n225 = property on="TAC Window" class="Bool"("Disabled"=w225) -> ()  [unwired: 2 in, 2 out]
                                }
                                }
                                }
                                frame #3 {
                                n226 = property on="Ampel" class="Clust (strict)"("Value"=cluster{"RED":bool, "RED 2":bool, "RED 3":bool} {"RED"=FALSE, "RED 2"=FALSE, "RED 3"=TRUE} ("Ampel")) -> ()  [unwired: 2 in, 2 out]
                                n227 = property on="Boolean" class="Bool (strict)"("Value"=TRUE) -> ()  [unwired: 2 in, 2 out]
                                n228 = property on="YELLOW" class="Bool (strict)"("Blinking"=FALSE) -> ()  [unwired: 2 in, 2 out]
                                }
                              }
                            }
                          }
                        }
                        frame #10 {
                          n229 = stacked-sequence {
                            frame #0 {
                              n230 = property on="Ampel" class="Clust (strict)"("Value"=cluster{"RED":bool, "YELLOW":bool, "GREEN":bool} {"RED"=FALSE, "YELLOW"=FALSE, "GREEN"=FALSE} ("Ampel")) -> ("Controls[]"=w235:refnum<vi>[])  [unwired: 2 in, 2 out]
                              n231 = Index Array(array=w235, index=1) -> (element=w233:refnum<vi>)
                              n232 = property class="Ctl"(reference=w233, "Blinking"=TRUE) -> ()  [unwired: 1 in, 2 out]
                            }
                            frame #1 {
                              n233 = control-ref of="plane"() -> (w241:refnum<vi>)
                              n234 = control-ref of="TACwinLoaded?"() -> (w243:refnum<vi>)
                              n235 = control-ref of="16btimage?"() -> (w242:refnum<vi>)
                              n236 = control-ref of="router"() -> (w240:refnum<vi>)
                              n237 = control-ref of="Image Path"() -> (w244:refnum<vi>)
                              n238 = control-ref of="notes"() -> (w239:refnum<vi>)
                              n239 = local read "first scan?"() -> (w237:bool)
                              n240 = control-ref of="Int duplex?"() -> (w245:refnum<vi>)
                              n241 = call "SpotFinder.vi"("first scan?"=w237, "auto"=TRUE, "Int duplex?"=w245, "notes"=w239, "router 3"=w240, "plane 2"=w241, "Image Path"=w244, "16bit?"=w242, "TACwinLoaded?"=w243) -> ()  [unwired: 2 in]
                            }
                            frame #2 {
                              n242 = control-ref of="Image Path"() -> (w247:refnum<vi>)
                              n243 = control-ref of="notes"() -> (w246:refnum<vi>)
                              n244 = call "SaveNotes.vi"("Enum"=enum16{"Get Path", "Read", "Save"}."Save", "String"=w246, "Path"=w247) -> ()  [unwired: 2 in]
                              n245 = property on="Ampel" class="Clust (strict)"("Value"=cluster{"RED":bool, "YELLOW":bool, "GREEN":bool} {"RED"=FALSE, "YELLOW"=FALSE, "GREEN"=TRUE} ("Ampel")) -> ("Controls[]"=w254:refnum<vi>[])  [unwired: 2 in, 2 out]
                              n246 = Index Array(array=w254, index=1) -> (element=w252:refnum<vi>)
                              n247 = property class="Ctl"(reference=w252, "Blinking"=FALSE) -> ()  [unwired: 1 in, 2 out]
                              n248 = local write "16btimage?"(FALSE ("16btimage?")) -> ()
                              n249 = local write "first scan?"(FALSE ("first scan?")) -> ()
                            }
                          }
                        }
                        frame #11 {
                          # "next file"
                          n250 = Strip Path(path=w260) -> (stripped path=w272:path, name=w269:string)
                          n251 = flat-sequence {
                            tunnel: [w276] -> w256
                            frame #0 {
                              n252 = property on="stop batch" class="Bool (strict)"("Visible"=TRUE, "DisabledEnum"=T6."Enabled" ("Disabled")) -> ()  [unwired: 2 in, 2 out]
                            }
                            frame #1 {
                              n253 = Wait (ms)(milliseconds to wait=u32 2000) -> ()  [unwired: 1 out]
                            }
                            frame #2 {
                              n254 = property on="stop batch" class="Bool (strict)"("Visible"=FALSE) -> ("Value"=w276:bool)  [unwired: 2 in, 2 out]
                            }
                            frame #3 {
                              n255 = property on="stop batch" class="Bool (strict)"("Value"=FALSE ("stop batch")) -> ()  [unwired: 2 in, 2 out]
                            }
                          }
                          n256 = Strip Path(path=w272) -> (stripped path=w266:path, name=w268:string)
                          n257 = Scan From String(format string="%d", input string=w268) -> (output 1=w270:i32)  [unwired: 3 in, 3 out]
                          n258 = Increment(x=w270) -> (x+1=w267:i32)
                          n259 = Number To Decimal String(number=w267) -> (decimal integer string=w265:string)  [unwired: 1 in]
                          n260 = Search and Replace String(input string=w269, search string=w268, replace string=w265) -> (result string=w263:string)  [unwired: 5 in, 3 out]
                          n261 = Not(x=w256) -> (.not. x?=w257:bool)
                          n262 = Build Path(base path=w266, name or relative path=w265) -> (appended path=w264:path)
                          n263 = Build Path(base path=w264, name or relative path=w263) -> (appended path=w261:path)
                          n264 = call <vilib>:"Check if File or Folder Exists.vi"("path"=w261) -> ("file or folder exists?"=w258:bool)  [unwired: 8 in, 2 out]
                          n265 = And(x=w258, y=w257) -> (x .and. y?=w259:bool)
                          n266 = call "FilePathGlobal.vi"("Image Path"=w261, "set?"=TRUE) -> ()  [unwired: 3 out]
                          n267 = local write "Image Path"(w261) -> ()
                        }
                      }
                    }
                  }
                }
              }
              frame #2 {
                n268 = property on="Batch Analyze" class="Bool"("Visible"=TRUE) -> ()  [unwired: 2 in, 2 out]
              }
            }
          }
          event #3 {
            n269 = event-data() -> ()  [unwired: 1 in, 5 out]
            n270 = stacked-sequence {
              seq-local: [_ w283 _] -> [_ _ w304]
              frame #0 {
              }
              frame #1 {
                n271 = while {
                  shift-right: [w286] -> w282
                  shift-left: "Image Path" -> [w287]
                  tunnel: [w285] -> w283
                  stop <- w288 stop-if-true
                  n272 = control-ref of="Image Path"() -> (w293:refnum<vi>)
                  n273 = Path To String(path=w287) -> (string=w290:string)
                  n274 = call "LoadHeaderKenandHerty.vi"("appended path"=w287, "reference"=w293) -> ("unsuccesful?"=w289:bool)  [unwired: 3 in]
                  n275 = Concatenate Strings("Anna_linescan " ("string"), w290) -> (w292:string)
                  n276 = property class="VI"("Front Panel Window:Title"=w292) -> ()  [unwired: 2 in, 2 out]
                  n277 = case shown="False" w289 {
                    tunnel: w287 -> [w294 w303]
                    tunnel: [TRUE w299] -> w288
                    tunnel: [w294 w301] -> w286
                    tunnel: [1 0] -> w285
                    frame #0 {
                    }
                    frame #1 {
                      (unwired) T10."existing file" ("select mode (2)")
                      n278 = File Dialog(6:"*.hd2; *.hdr; fileinfo.txt" ("pattern"), 7:"Select Header File" ("prompt"), 11:w303) -> (0:w297:errorcluster, 1:w299:bool, 3:w301:path)  [unwired: 4 in, 1 out]
                      n279 = Unbundle(w297) -> ()  [unwired: 3 out]
                    }
                  }
                }
                n280 = call "FilePathGlobal.vi"("Image Path"=w282, "set?"=TRUE) -> ()  [unwired: 3 out]
              }
              frame #2 {
                n281 = for {
                  N: w304 -> [_]
                  n282 = stacked-sequence {
                    frame #0 {
                      w306 = u8 2 ("Disabled")
                      w305 = FALSE ("Boolean")
                      n283 = property on="Image LOADED" class="Boolean (strict)"("Value"=w305, "Blinking"=w305) -> ()  [unwired: 2 in, 2 out]
                      n284 = property on="Spotfinder" class="Boolean"("Disabled"=w306) -> ()  [unwired: 2 in, 2 out]
                      n285 = property on="TAC Window" class="Boolean"("Disabled"=w306) -> ()  [unwired: 2 in, 2 out]
                      n286 = property on="Export" class="Boolean"("Disabled"=w306) -> ()  [unwired: 2 in, 2 out]
                      n287 = property on="View Image Settings" class="Boolean"("Disabled"=w306) -> ()  [unwired: 2 in, 2 out]
                      n288 = property on="View FIFO Settings" class="Boolean"("Disabled"=w306) -> ()  [unwired: 2 in, 2 out]
                    }
                    frame #1 {
                      n289 = call "ViewImageSetnew.vi"("action"=enum16{"Display", "change", "Get", "Set"}."Get" ("Enum")) -> ("Image Settings"=w308:T11)  [unwired: 2 in]
                      n290 = Unbundle By Name(w308) -> ("Retrace"=w307:bool)
                      n291 = case shown="False" w307 {
                        frame #0 {
                          n292 = property on="Load Image" class="Boolean"("Disabled"=u8 0, "Visible"=TRUE) -> ()  [unwired: 2 in, 2 out]
                        }
                        frame #1 {
                          n293 = property on="Load Image" class="Boolean"("Disabled"=u8 2, "Visible"=FALSE) -> ()  [unwired: 2 in, 2 out]
                          n294 = One Button Dialog(message="Die Retrace kann derzeit noch nicht bearbeitet werden.") -> ()  [unwired: 1 in, 1 out]
                        }
                      }
                    }
                    frame #2 {
                      n295 = control-ref of="notes"() -> (w317:refnum<vi>)
                      n296 = control-ref of="Image Path"() -> (w315:refnum<vi>)
                      n297 = call "SaveNotes.vi"("Enum"=enum16{"Get Path", "Read", "Save"}."Get Path", "String"=w317, "Path"=w315) -> ()  [unwired: 2 in]
                    }
                    frame #3 {
                      w320 = u8 0 ("Disabled")
                      n298 = property on="Load" class="Bool"("Visible"=FALSE) -> ()  [unwired: 2 in, 2 out]
                      n299 = property on="Image LOADED" class="Boolean (strict)"("Disabled"=w320) -> ()  [unwired: 2 in, 2 out]
                      n300 = property on="View Image Settings" class="Boolean"("Disabled"=w320) -> ()  [unwired: 2 in, 2 out]
                      n301 = property on="View FIFO Settings" class="Boolean"("Disabled"=w320) -> ()  [unwired: 2 in, 2 out]
                      n302 = property on="LOADED HDR" class="Bool (strict)"("Value"=TRUE ("Boolean")) -> ()  [unwired: 2 in, 2 out]
                      n303 = property on="Ampel" class="Clust (strict)"("Value"=cluster{"RED":bool, "RED 2":bool, "RED 3":bool} {"RED"=TRUE, "RED 2"=TRUE, "RED 3"=FALSE} ("Ampel")) -> ()  [unwired: 2 in, 2 out]
                    }
                  }
                }
              }
            }
          }
          event #4 {
            n304 = event-data() -> ()  [unwired: 1 in, 5 out]
            n305 = stacked-sequence {
              frame #0 {
              }
              frame #1 {
                n306 = property on="Image LOADED" class="Boolean (strict)"("Blinking"=TRUE) -> ()  [unwired: 2 in, 2 out]
                n307 = property on="Image Path" class="Path"("Disabled"=u8 2) -> ()  [unwired: 2 in, 2 out]
                n308 = property on="Load Image" class="Boolean"("Disabled"=u8 2) -> ()  [unwired: 2 in, 2 out]
                n309 = call "sumofphotons.vi"("s"=TRUE, "sum of photons"=u32[][][][] []) -> ()  [unwired: 1 out]
              }
              frame #2 {
                n310 = call "WriteTempData.vi"("Enum"=enum16{"create new", "write", "close"}."create new") -> ("error out"=w328:errorcluster)  [unwired: 4 in, 1 out]
                n311 = call "HandleError.vi"("error in (no error)"=w328) -> ()
              }
              frame #3 {
                n312 = call "fileformatGlobal.vi"("changed"=FALSE) -> ("fileformat out"=w330:enum16{"Herty", "Ken", "SPC130", "HydraHarp"})  [unwired: 1 in]
                n313 = control-ref of="Image Path"() -> (w332:refnum<vi>)
                n314 = case shown="\"Herty\", Default" w330 {
                  tunnel: w332 -> [w333 w334 w335 w336]
                  frame #0 {
                    n315 = call "LoadData.vi"("Path"=w333) -> ()  [unwired: 2 in, 3 out]
                  }
                  frame #1 {
                    n316 = call "LoadDataSPC130.vi"("Path"=w334) -> ()  [unwired: 2 in, 3 out]
                  }
                  frame #2 {
                    n317 = call "LoadDataHH.vi"("Path"=w335) -> ()  [unwired: 2 in, 3 out]
                  }
                  frame #3 {
                    n318 = call "LoadDataKen.vi"("Path"=w336) -> ()  [unwired: 5 in]
                  }
                }
              }
              frame #4 {
                n319 = call "WriteTempData.vi"("Enum"=enum16{"create new", "write", "close"}."close") -> ("error out"=w337:errorcluster)  [unwired: 4 in, 1 out]
                n320 = call "HandleError.vi"("error in (no error)"=w337) -> ()
              }
              frame #5 {
                n321 = call "TotalRecall_Reload.vi"() -> ("gap"=→"gap":i32, "invalid"=→"invalid":i32, "valid"=→"total":i32)  [unwired: 4 in, 1 out]
              }
              frame #6 {
                n322 = call "ViewFIFOSet.vi"("Enum"=T5."Get") -> ("FIFO Settings (Array)"=w348:T12[])  [unwired: 1 in]
                n323 = Index Array(array=w348) -> (element=w349:T12)  [unwired: 1 in]
                n324 = Array Size(array=w348) -> (size(s)=w344:i32)
                n325 = Unbundle By Name(w349) -> ("Measurement.No of Channels"=w343:u16)
                n326 = Multiply(x=w343, y=w344) -> (x*y=w342:i32)
                n327 = for {
                  N: w342 -> [_]
                  tunnel: [w358] -> w347 mode=indexing
                  i -> [w359]
                  n328 = Number To Decimal String(number=w359) -> (decimal integer string=w358:string)  [unwired: 1 in]
                }
                n329 = Build Array (concatenate)("sum", w347) -> (w345:string[])
                n330 = property on="router" class="Ring (strict)"("Strings []"=w345) -> ("Value"=w354:u8)  [unwired: 2 in, 2 out]
                n331 = property on="plane" class="DigNum (strict)"() -> ("Value"=w355:u32)  [unwired: 2 in, 2 out]
                n332 = property on="threshold" class="Clust (strict)"() -> ("Value"=w351:cluster{"max":u32, "min":u32})  [unwired: 2 in, 2 out]
                n333 = call "sumofphotons.vi"("s"=FALSE) -> ("sum of photons out"=w352:u32[][][][])  [unwired: 1 in]
                n334 = property on="RGB or false color?" class="Bool (strict)"() -> ("Value"=w356:bool)  [unwired: 2 in, 2 out]
                n335 = call "OnlinePic.vi"("action"=T2."ini" ("Enum"), "RGB/False"=w356, "Threshold (max)"=w351, "plane"=w355, "router channel"=w354, "Array"=w352) -> ()  [unwired: 1 in, 5 out]
              }
              frame #7 {
                n336 = call "ViewImageSetnew.vi"("action"=enum16{"Display", "change", "Get", "Set"}."Get" ("Enum")) -> ("Image Settings"=w361:T11)  [unwired: 2 in]
                n337 = Unbundle By Name(w361) -> ("Image Size (pixel).z"=w362:u32)
                n338 = case shown="0" w362 {
                  tunnel: [i8 2 w367] -> w363
                  tunnel: [u8 0 w367] -> w364
                  frame #0 {
                  }
                  frame #1 {
                    w367 = u8 0
                  }
                }
                n339 = property on="plane" class="DigNum (strict)"("Disabled"=w363, "Value"=w364) -> ()  [unwired: 2 in, 2 out]
              }
              frame #8 {
                w368 = u8 0
                n340 = property on="Image LOADED" class="Boolean (strict)"("Blinking"=FALSE, "Value"=TRUE ("Image LOADED")) -> ()  [unwired: 2 in, 2 out]
                n341 = property on="Lifetime pick" class="Boolean"("Disabled"=w368) -> ()  [unwired: 2 in, 2 out]
                n342 = property on="RGB or false color?" class="Boolean (strict)"("Disabled"=w368) -> ()  [unwired: 2 in, 2 out]
                n343 = property on="16bit" class="Boolean"("Disabled"=w368) -> ()  [unwired: 2 in, 2 out]
                n344 = property on="threshold" class="Clust (strict)"("Disabled"=w368) -> ()  [unwired: 2 in, 2 out]
                n345 = property on="Spotfinder" class="Boolean"("Disabled"=w368) -> ()  [unwired: 2 in, 2 out]
                n346 = property on="router" class="Ring (strict)"("Disabled"=w368) -> ()  [unwired: 2 in, 2 out]
                n347 = property on="coincidence spot" class="Boolean"("Disabled"=w368) -> ()  [unwired: 2 in, 2 out]
                n348 = property on="TAC Window" class="Boolean"("Disabled"=w368) -> ()  [unwired: 2 in, 2 out]
                n349 = property on="Export" class="Bool"("Disabled"=w368) -> ()  [unwired: 2 in, 2 out]
                n350 = property on="F2-Image" class="Boolean"("Disabled"=u8 0) -> ()  [unwired: 2 in, 2 out]
                n351 = property on="coincidence\nimage" class="Bool"("Disabled"=w368) -> ()  [unwired: 2 in, 2 out]
              }
              frame #9 {
                n352 = property on="Ampel" class="Clust (strict)"("Value"=cluster{"RED":bool, "RED 2":bool, "RED 3":bool} {"RED"=FALSE, "RED 2"=FALSE, "RED 3"=TRUE} ("Ampel")) -> ()  [unwired: 2 in, 2 out]
              }
            }
          }
          event #5 {
            n353 = event-data() -> ()  [unwired: 1 in, 5 out]
            n354 = Unbundle By Name("threshold") -> ("max"=w378:u32, "min"=w377:u32)
            n355 = call "CheckPlane.vi"("plane 2"="plane") -> ("plane"=w379:u32)
            n356 = Max & Min(x=w378, y=w377) -> (max(x,y)=w376:u32, min(x,y)=w375:u32)
            n357 = Bundle By Name(cluster="threshold", "max"=w376, "min"=w375) -> (w373:cluster{"max":u32, "min":u32})
            n358 = property on="threshold" class="Cluster (strict)"("Value"=w373) -> ()  [unwired: 2 in, 2 out]
            n359 = property on="plane" class="DigNum (strict)"("Value"=w379) -> ()  [unwired: 2 in, 2 out]
            n360 = property on="16btimage?" class="Bool (strict)"() -> ("Value"=w388:bool)  [unwired: 2 in, 2 out]
            n361 = call "OnlinePic.vi"("action"=T2."Change" ("Enum"), "RGB/False"="RGB or false color?", "Threshold (max)"=w373, "plane"=w379, "router channel"="router") -> ()  [unwired: 2 in, 5 out]
            n362 = call "StandardSettings.vi"("Enum"=enum16{"Load", "get", "Save", "set"}."get") -> ("StandardSettings"=w384:T9)  [unwired: 4 in]
            n363 = Bundle By Name(cluster=w384, "threshold"=w373, "RGB or false color"="RGB or false color?") -> (w383:T9)
            n364 = case shown="True" w388 {
              tunnel: "router" -> [_ w393]
              tunnel: w379 -> [_ w392]
              frame #0 {
              }
              frame #1 {
                n365 = call "16bitImageglobal.vi"("Enum"=T4."Input", "plane"=w392, "router"=w393) -> ("error out"=w390:errorcluster)  [unwired: 2 in, 3 out]
                n366 = call "HandleError.vi"("error in (no error)"=w390) -> ()
              }
            }
            n367 = call "StandardSettings.vi"("StandardSettings"=w383, "Enum"=enum16{"Load", "get", "Save", "set"}."set") -> ()  [unwired: 3 in, 1 out]
          }
          event #6 {
            n368 = event-data() -> ()  [unwired: 1 in, 5 out]
            n369 = stacked-sequence {
              seq-local: [_ _ _ w424 _] -> [_ _ _ _ w429]
              frame #0 {
                n370 = property on="Ampel" class="Clust (strict)"("Value"=cluster{"RED":bool, "RED 2":bool, "RED 3":bool} {"RED"=FALSE, "RED 2"=FALSE, "RED 3"=FALSE} ("Ampel")) -> ()  [unwired: 2 in, 2 out]
                n371 = property on="TACwinLoaded?" class="Boolean (strict)"() -> ("Value"=w399:bool)  [unwired: 2 in, 2 out]
                n372 = call "Intensityduplex.vi"("Enum"=T3."dump") -> ()  [unwired: 4 in, 2 out]
                n373 = case shown="False" w399 {
                  frame #0 {
                    n374 = call "GetTACWindow.vi"("Enum"=enum16{"ini", "get", "quick"}."quick") -> ()  [unwired: 1 in, 9 out]
                  }
                  frame #1 {
                  }
                }
                n375 = property on="YELLOW" class="Boolean (strict)"("Blinking"=TRUE) -> ()  [unwired: 2 in, 2 out]
              }
              frame #1 {
                n376 = property on="threshold" class="Clust (strict)"() -> ("Value"=w401:cluster{"max":u32, "min":u32})  [unwired: 2 in, 2 out]
                n377 = call "StandardSettings.vi"("Enum"=enum16{"Load", "get", "Save", "set"}."get") -> ("StandardSettings"=w403:T9)  [unwired: 4 in]
                n378 = Bundle By Name(cluster=w403, "threshold"=w401) -> (w402:T9)
                n379 = property on="notes" class="String"() -> ("Value"=w407:string)  [unwired: 2 in, 2 out]
                n380 = Concatenate Strings(w407, "\n- lifetime picking" ("string")) -> (w406:string)
                n381 = call "StandardSettings.vi"("StandardSettings"=w402, "Enum"=enum16{"Load", "get", "Save", "set"}."set") -> ()  [unwired: 3 in, 1 out]
                n382 = control-ref of="Image Path"() -> (w411:refnum<vi>)
                n383 = property on="notes" class="String"("Value"=w406) -> ()  [unwired: 2 in, 2 out]
                n384 = call "WriteStoreData.vi"("Enum"=enum16{"Save", "Control"}."Control", "Image Path"=w411) -> ("already x spots"=→"already x spots":i16)  [unwired: 1 in]
              }
              frame #2 {
                n385 = property on="already x spots" class="Digital (strict)"() -> ("Value"=w414:i16)  [unwired: 2 in, 2 out]
                n386 = control-ref of="notes"() -> (w413:refnum<vi>)
                n387 = call "LifetimePickTACCube.vi"("notes 2"=w413, "already x spots"=w414) -> ("spots"=→"spots":i16)  [unwired: 1 in]
              }
              frame #3 {
                w423 = "%02d to %02d" ("format string")
                n388 = property on="already x spots" class="Digital (strict)"() -> ("Value"=w422:i16)  [unwired: 2 in, 2 out]
                n389 = property on="spots" class="Digital (strict)"() -> ("Value"=w421:i16)  [unwired: 2 in, 2 out]
                n390 = Greater?(x=w422, y=w421) -> (0:w420:bool)
                n391 = Decrement(x=w421) -> (x-1=w425:i16)
                n392 = Format Into String(format string=w423, initial string=" spots ", w422, w425) -> ()  [unwired: 1 in, 2 out]
                n393 = Format Into String(format string=w423, w422, w425) -> (resulting string=w424:string)  [unwired: 2 in, 1 out]
                n394 = Select(t=w423, s=w420, f="") -> (s? t:f=w418:string)
                n395 = call "Intensityduplex.vi"("Enum"=T3."name", "add string"=w418) -> ()  [unwired: 3 in, 2 out]
                n396 = call "OnlinePic.vi"("action"=T2."Get" ("Enum")) -> ("RGB/False out"=w416:bool, "Threshold (max) OUT"=w415:cluster{"max":u32, "min":u32})  [unwired: 6 in, 3 out]
                n397 = property on="RGB or false color?" class="Bool (strict)"("Value"=w416) -> ()  [unwired: 2 in, 2 out]
                n398 = property on="threshold" class="Clust (strict)"("Value"=w415) -> ()  [unwired: 2 in, 2 out]
              }
              frame #4 {
                n399 = call "StoreDatafromLifetimePick.vi"("Enum"=enum16{"clear", "Get", "Set", "Add"}."Get") -> ("Spots"=w428:T13[], "store s.th.?"=w433:bool)  [unwired: 1 in]
                n400 = case shown="True" w433 {
                  tunnel: w429 -> [_ w436]
                  tunnel: w428 -> [_ w435]
                  frame #0 {
                  }
                  frame #1 {
                    n401 = stacked-sequence {
                      tunnel: w436 -> [_ w441]
                      tunnel: w435 -> [w437 _]
                      frame #0 {
                        n402 = control-ref of="Image Path"() -> (w439:refnum<vi>)
                        n403 = call "WriteStoreData.vi"("Spots"=w437, "Enum"=enum16{"Save", "Control"}."Save", "Image Path"=w439) -> ()  [unwired: 1 out]
                      }
                      frame #1 {
                        n404 = property on="notes" class="String"() -> ("Value"=w443:string)  [unwired: 2 in, 2 out]
                        n405 = Concatenate Strings(w443, "\npick result spots (" ("string"), w441, ") and decays stored in IMAGE PATH\n" ("string")) -> (w442:string)
                        n406 = property on="notes" class="String"("Value"=w442) -> ()  [unwired: 2 in, 2 out]
                      }
                    }
                  }
                }
                n407 = property on="Int duplex?" class="Boolean (strict)"("Value"=TRUE ("Boolean 2")) -> ()  [unwired: 2 in, 2 out]
                n408 = property on="Ampel" class="Clust (strict)"("Value"=cluster{"RED":bool, "RED 2":bool, "RED 3":bool} {"RED"=FALSE, "RED 2"=FALSE, "RED 3"=TRUE} ("Ampel")) -> ()  [unwired: 2 in, 2 out]
                n409 = property on="YELLOW" class="Boolean (strict)"("Blinking"=FALSE) -> ()  [unwired: 2 in, 2 out]
              }
            }
          }
          event #7 {
            n410 = event-data() -> ()  [unwired: 1 in, 5 out]
          }
          event #8 {
            n411 = event-data() -> ()  [unwired: 1 in, 5 out]
            n412 = stacked-sequence {
              frame #0 {
              }
              frame #1 {
                n413 = control-ref of="Image Path"() -> (w447:refnum<vi>)
                n414 = call "GetSetTempDir.vi"("Path"=w447) -> ()  [unwired: 4 in]
              }
            }
          }
          event #9 {
            n415 = event-data() -> ()  [unwired: 1 in, 5 out]
            n416 = stacked-sequence {
              frame #0 {
                n417 = property on="Ampel" class="Clust (strict)"("Value"=cluster{"RED":bool, "RED 2":bool, "RED 3":bool} {"RED"=FALSE, "RED 2"=FALSE, "RED 3"=FALSE} ("Ampel")) -> ()  [unwired: 2 in, 2 out]
                n418 = property on="YELLOW" class="Boolean (strict)"("Blinking"=TRUE) -> ()  [unwired: 2 in, 2 out]
              }
              frame #1 {
                n419 = property on="Image LOADED" class="Bool (strict)"() -> ("Value"=w451:bool)  [unwired: 2 in, 2 out]
                n420 = case shown="True" w451 {
                  frame #0 {
                  }
                  frame #1 {
                    n421 = call "GetTACWindow.vi"("Enum"=enum16{"ini", "get", "quick"}."ini") -> ("Cursor.Cursor Position:Cursor X"=w460:u16, "Cursor.Cursor Position:Cursor X 2"=w461:u16, "x-values"=w454:dbl[], "ready?"=w455:bool)  [unwired: 1 in, 5 out]
                    n422 = Select(t=2, s=w455, f=0) -> (s? t:f=w458:i32)
                    n423 = property on="TACwinLoaded?" class="Boolean (strict)"("Value"=TRUE ("TACwinLoaded?")) -> ()  [unwired: 2 in, 2 out]
                    n424 = call "CursorPositionChanged.vi"("CursorPos x1"=w461, "CursorPos x0"=w460, "x-values"=w454, "action"=enum16{"Check", "Get", "xval"}."xval" ("Enum")) -> ()  [unwired: 4 out]
                    n425 = property on="TAC Window" class="Boolean"("Disabled"=w458) -> ()  [unwired: 2 in, 2 out]
                  }
                }
              }
              frame #2 {
                n426 = property on="Ampel" class="Clust (strict)"("Value"=cluster{"RED":bool, "RED 2":bool, "RED 3":bool} {"RED"=FALSE, "RED 2"=FALSE, "RED 3"=TRUE} ("Ampel")) -> ()  [unwired: 2 in, 2 out]
                n427 = property on="YELLOW" class="Boolean (strict)"("Blinking"=FALSE) -> ()  [unwired: 2 in, 2 out]
                "Boolean" <- TRUE
              }
            }
          }
          event #10 {
            n428 = event-data() -> ()  [unwired: 1 in, 5 out]
            n429 = stacked-sequence {
              frame #0 {
                n430 = property on="Ampel" class="Clust (strict)"("Value"=cluster{"RED":bool, "YELLOW":bool, "GREEN":bool} {"RED"=FALSE, "YELLOW"=FALSE, "GREEN"=FALSE} ("Ampel")) -> ("Controls[]"=w469:refnum<vi>[])  [unwired: 2 in, 2 out]
                n431 = Index Array(array=w469, index=1) -> (element=w467:refnum<vi>)
                n432 = property class="Ctl"(reference=w467, "Blinking"=TRUE) -> ()  [unwired: 1 in, 2 out]
              }
              frame #1 {
                n433 = control-ref of="plane"() -> (w475:refnum<vi>)
                n434 = control-ref of="TACwinLoaded?"() -> (w477:refnum<vi>)
                n435 = control-ref of="16btimage?"() -> (w476:refnum<vi>)
                n436 = control-ref of="router"() -> (w474:refnum<vi>)
                n437 = control-ref of="Image Path"() -> (w478:refnum<vi>)
                n438 = control-ref of="notes"() -> (w473:refnum<vi>)
                n439 = control-ref of="Int duplex?"() -> (w479:refnum<vi>)
                n440 = call "SpotFinder.vi"("first scan?"=TRUE, "auto"=FALSE, "Int duplex?"=w479, "notes"=w473, "router 3"=w474, "plane 2"=w475, "Image Path"=w478, "16bit?"=w476, "TACwinLoaded?"=w477) -> ()  [unwired: 2 in]
              }
              frame #2 {
                n441 = property on="Ampel" class="Clust (strict)"("Value"=cluster{"RED":bool, "YELLOW":bool, "GREEN":bool} {"RED"=FALSE, "YELLOW"=FALSE, "GREEN"=TRUE} ("Ampel")) -> ("Controls[]"=w483:refnum<vi>[])  [unwired: 2 in, 2 out]
                n442 = Index Array(array=w483, index=1) -> (element=w481:refnum<vi>)
                n443 = property class="Ctl"(reference=w481, "Blinking"=FALSE) -> ()  [unwired: 1 in, 2 out]
              }
            }
          }
          event #11 {
            n444 = event-data() -> ()  [unwired: 1 in, 5 out]
            n445 = stacked-sequence {
              frame #0 {
              }
              frame #1 {
                n446 = control-ref of="Int duplex?"() -> (w490:refnum<vi>)
                n447 = control-ref of="16btimage?"() -> (w489:refnum<vi>)
                n448 = control-ref of="does a coinc image exist?"() -> (w488:refnum<vi>)
                n449 = control-ref of="Image Path"() -> (w487:refnum<vi>)
                n450 = control-ref of="notes"() -> (w486:refnum<vi>)
                n451 = call "ExportDialog.vi"("Int duplex ctl"=w490, "16 bit ctl"=w489, "coincidence image ctl"=w488, "Path"=w487, "notes 2"=w486) -> ()  [unwired: 4 in]
              }
            }
          }
          event #12 {
            n452 = event-data() -> ()  [unwired: 1 in, 5 out]
            n453 = stacked-sequence {
              frame #0 {
                n454 = property on="Ampel" class="Clust (strict)"("Value"=cluster{"RED":bool, "RED 2":bool, "RED 3":bool} {"RED"=FALSE, "RED 2"=FALSE, "RED 3"=FALSE} ("Ampel")) -> ()  [unwired: 2 in, 2 out]
                n455 = property on="YELLOW" class="Boolean (strict)"("Blinking"=TRUE) -> ()  [unwired: 2 in, 2 out]
              }
              frame #1 {
                n456 = property on="TACwinLoaded?" class="Bool (strict)"() -> ("Value"=w494:bool)  [unwired: 2 in, 2 out]
                n457 = case shown="False" w494 {
                  frame #0 {
                    n458 = call "GetTACWindow.vi"("Enum"=enum16{"ini", "get", "quick"}."ini") -> ("Cursor.Cursor Position:Cursor X"=w498:u16, "Cursor.Cursor Position:Cursor X 2"=w497:u16, "x-values"=w496:dbl[])  [unwired: 1 in, 6 out]
                    n459 = call "CursorPositionChanged.vi"("CursorPos x1"=w497, "CursorPos x0"=w498, "x-values"=w496, "action"=enum16{"Check", "Get", "xval"}."xval" ("Enum")) -> ()  [unwired: 4 out]
                  }
                  frame #1 {
                  }
                }
              }
              frame #2 {
                n460 = property on="notes" class="String"() -> ("Value"=w501:string)  [unwired: 2 in, 2 out]
                n461 = Concatenate Strings(w501, "\n- F2 and lifetime image" ("string")) -> (w500:string)
                n462 = property on="notes" class="String"("Value"=w500) -> ()  [unwired: 2 in, 2 out]
              }
              frame #3 {
                n463 = property on="threshold" class="Clust (strict)"() -> ("Value"=w506:cluster{"max":u32, "min":u32})  [unwired: 2 in, 2 out]
                n464 = control-ref of="notes"() -> (w507:refnum<vi>)
                n465 = Unbundle(w506) -> ("max"=w505:u32, "min"=w504:u32)
                n466 = Max & Min(x=w505, y=w504) -> (min(x,y)=w503:u32)  [unwired: 1 out]
                n467 = control-ref of="Image Path"() -> (w508:refnum<vi>)
                n468 = call "ShowLifetimeAndF2Image.vi"("Path"=w508, "threshold (min)"=w503, "notes 2"=w507) -> ()  [unwired: 4 in]
              }
              frame #4 {
                n469 = property on="Ampel" class="Clust (strict)"("Value"=cluster{"RED":bool, "RED 2":bool, "RED 3":bool} {"RED"=FALSE, "RED 2"=FALSE, "RED 3"=TRUE} ("Ampel")) -> ()  [unwired: 2 in, 2 out]
                n470 = property on="YELLOW" class="Boolean (strict)"("Blinking"=FALSE) -> ()  [unwired: 2 in, 2 out]
              }
            }
          }
          event #13 {
            n471 = event-data() -> ()  [unwired: 1 in, 5 out]
            n472 = stacked-sequence {
              frame #0 {
                n473 = property on="16btimage?" class="Boolean (strict)"() -> ("Value"=w513:bool)  [unwired: 2 in, 2 out]
                n474 = Not(x=w513) -> (.not. x?=→"16btimage?":bool)
              }
              frame #1 {
                n475 = property on="16btimage?" class="Boolean (strict)"() -> ("Value"=w514:bool)  [unwired: 2 in, 2 out]
                n476 = case shown="True" w514 {
                  frame #0 {
                    n477 = call "16bitImageglobal.vi"("Enum"=T4."Dump") -> ()  [unwired: 4 in, 4 out]
                  }
                  frame #1 {
                    n478 = stacked-sequence {
                      frame #0 {
                        n479 = call "16bitImageglobal.vi"("Enum"=T4."Ini") -> ()  [unwired: 4 in, 4 out]
                      }
                      frame #1 {
                        n480 = property on="router" class="Ring (strict)"() -> ("Value"=w519:u8)  [unwired: 2 in, 2 out]
                        n481 = property on="plane" class="DigNum (strict)"() -> ("Value"=w518:u32)  [unwired: 2 in, 2 out]
                        n482 = call "16bitImageglobal.vi"("Enum"=T4."Input", "plane"=w518, "router"=w519) -> ()  [unwired: 2 in, 4 out]
                      }
                      frame #2 {
                        n483 = call "16bitImageglobal.vi"("Enum"=T4."Get") -> ()  [unwired: 4 in, 4 out]
                      }
                    }
                  }
                }
              }
            }
          }
          event #14 {
            n484 = event-data() -> ()  [unwired: 1 in, 5 out]
            n485 = stacked-sequence {
              frame #0 {
                n486 = property on="Ampel" class="Clust (strict)"("Value"=cluster{"RED":bool, "RED 2":bool, "RED 3":bool} {"RED"=FALSE, "RED 2"=FALSE, "RED 3"=FALSE} ("Ampel")) -> ()  [unwired: 2 in, 2 out]
                n487 = property on="YELLOW" class="Boolean (strict)"("Blinking"=TRUE) -> ()  [unwired: 2 in, 2 out]
                n488 = call "Intensityduplex.vi"("Enum"=T3."dump") -> ()  [unwired: 4 in, 2 out]
              }
              frame #1 {
                n489 = property on="notes" class="String"() -> ("Value"=w526:string)  [unwired: 2 in, 2 out]
                n490 = Concatenate Strings(w526, "\n- coincidence spotting" ("string")) -> (w525:string)
                n491 = property on="notes" class="String"("Value"=w525) -> ()  [unwired: 2 in, 2 out]
              }
              frame #2 {
                n492 = control-ref of="notes"() -> (w528:refnum<vi>)
                n493 = call "coincidenceImagenew.vi"("notes 2"=w528) -> ()  [unwired: 6 in]
              }
              frame #3 {
                n494 = property on="Ampel" class="Clust (strict)"("Value"=cluster{"RED":bool, "RED 2":bool, "RED 3":bool} {"RED"=FALSE, "RED 2"=FALSE, "RED 3"=TRUE} ("Ampel")) -> ()  [unwired: 2 in, 2 out]
                n495 = property on="YELLOW" class="Boolean (strict)"("Blinking"=FALSE) -> ()  [unwired: 2 in, 2 out]
              }
            }
          }
          event #15 {
            n496 = event-data() -> ()  [unwired: 1 in, 5 out]
            n497 = stacked-sequence {
              frame #0 {
                n498 = call "CoincidencePicture.vi"("Enum"=T7."Dump") -> ()  [unwired: 6 in, 3 out]
              }
              frame #1 {
                n499 = property on="notes" class="String"() -> ("Value"=w534:string)  [unwired: 2 in, 2 out]
                n500 = Concatenate Strings(w534, "\n- coincidence image" ("string")) -> (w533:string)
                n501 = property on="notes" class="String"("Value"=w533) -> ()  [unwired: 2 in, 2 out]
              }
              frame #2 {
                n502 = control-ref of="notes"() -> (w536:refnum<vi>)
                n503 = call "CoincidenceBuildImage.vi"("notes 2"=w536) -> ()  [unwired: 11 in]
              }
              frame #3 {
                n504 = call "CoincidencePicture.vi"("Enum"=enum16{"Ini", "Get", "Set", "Draw", "Colorpal"}."Get") -> ("String"=w539:string)  [unwired: 6 in, 2 out]
                n505 = Not Equal?(x=w539, y="") -> (x != y?=→"does a coinc image exist?":bool)
              }
            }
          }
          event #16 {
            n506 = event-data() -> ()  [unwired: 1 in, 5 out]
            n507 = stacked-sequence {
              frame #0 {
                n508 = call "ScanSubDirGlobal.vi"("set"=FALSE) -> ("Array"=w546:path[])  [unwired: 1 in]
                n509 = Index Array(array=w546, index="Header Path Ring") -> (element=w542:path)
                n510 = control-ref of="Image Path"() -> (w544:refnum<vi>)
                n511 = call "LoadHeaderKenandHerty.vi"("appended path"=w542, "reference"=w544) -> ("unsuccesful?"=w543:bool)  [unwired: 3 in]
                n512 = case shown="False" w543 {
                  tunnel: w542 -> [w548 _]
                  frame #0 {
                    n513 = call "FilePathGlobal.vi"("Image Path"=w548, "set?"=TRUE) -> ()  [unwired: 3 out]
                  }
                  frame #1 {
                  }
                }
              }
              frame #1 {
                n514 = control-ref of="notes"() -> (w550:refnum<vi>)
                n515 = control-ref of="Image Path"() -> (w552:refnum<vi>)
                n516 = call "SaveNotes.vi"("Enum"=enum16{"Get Path", "Read", "Save"}."Get Path", "String"=w550, "Path"=w552) -> ()  [unwired: 2 in]
              }
              frame #2 {
                w557 = u8 0 ("Disabled")
                n517 = property on="Load" class="Bool"("Visible"=FALSE) -> ()  [unwired: 2 in, 2 out]
                n518 = property on="Image LOADED" class="Boolean (strict)"("Disabled"=w557) -> ()  [unwired: 2 in, 2 out]
                n519 = property on="View Image Settings" class="Boolean"("Disabled"=w557) -> ()  [unwired: 2 in, 2 out]
                n520 = property on="View FIFO Settings" class="Boolean"("Disabled"=w557) -> ()  [unwired: 2 in, 2 out]
                n521 = property on="LOADED HDR" class="Bool (strict)"("Value"=TRUE ("Boolean")) -> ()  [unwired: 2 in, 2 out]
                n522 = property on="Ampel" class="Clust (strict)"("Value"=cluster{"RED":bool, "RED 2":bool, "RED 3":bool} {"RED"=TRUE, "RED 2"=TRUE, "RED 3"=FALSE} ("Ampel")) -> ()  [unwired: 2 in, 2 out]
                n523 = call "ViewImageSetnew.vi"("action"=enum16{"Display", "change", "Get", "Set"}."Get" ("Enum")) -> ("Image Settings"=w554:T11)  [unwired: 2 in]
                n524 = Unbundle By Name(w554) -> ("Retrace"=w555:bool)
                n525 = case shown="False" w555 {
                  frame #0 {
                    n526 = property on="Load Image" class="Boolean"("Disabled"=u8 0, "Visible"=TRUE) -> ()  [unwired: 2 in, 2 out]
                  }
                  frame #1 {
                    n527 = property on="Load Image" class="Boolean"("Disabled"=u8 2, "Visible"=FALSE) -> ()  [unwired: 2 in, 2 out]
                    n528 = One Button Dialog(message="Die Retrace kann derzeit noch nicht bearbeitet werden.") -> ()  [unwired: 1 in, 1 out]
                  }
                }
              }
              frame #3 {
                n529 = call "TempPath.vi"("change"=FALSE) -> ("stripped path 2"=w576:path)  [unwired: 2 in]
                n530 = Build Path(base path=w576, name or relative path="Anna_linescan.tmp" ("prompt")) -> (appended path=w574:path)
                n531 = property on="Image LOADED" class="Boolean (strict)"("Blinking"=TRUE) -> ()  [unwired: 2 in, 2 out]
                n532 = call <vilib>:"compatOverwrite.vi"("overwrite (F)"=TRUE) -> ("overwrite?"=w565:T14)
                n533 = Open/Create/Replace Datalog(5:T8 {"router"=[], "macro times"=[], "micro times"=[], "invalid"=[], "gap"=[]} ("cluster"), 10:w565, 11:w574) -> (3:w572:refnum<k1>)  [unwired: 3 in, 2 out]
                n534 = call "TempRefnum.vi"("change?"=TRUE, "refnum in"=w572) -> ()  [unwired: 1 out]
                n535 = property on="Header Path Ring" class="Ring (strict)"("Disabled"=u8 2) -> ()  [unwired: 2 in, 2 out]
                n536 = property on="Load Image" class="Boolean"("Disabled"=u8 2) -> ()  [unwired: 2 in, 2 out]
                n537 = call "sumofphotons.vi"("s"=TRUE, "sum of photons"=u32[][][][] []) -> ()  [unwired: 1 out]
              }
              frame #4 {
                n538 = control-ref of="Image Path"() -> (w579:refnum<vi>)
                n539 = call "fileformatGlobal.vi"("changed"=FALSE) -> ("fileformat out"=w581:enum16{"Herty", "Ken", "SPC130", "HydraHarp"})  [unwired: 1 in]
                n540 = case shown="\"Ken\"" w581 {
                  tunnel: w579 -> [w582 w583 w584]
                  frame #0 {
                    n541 = call "LoadData.vi"("Path"=w582) -> ()  [unwired: 2 in, 3 out]
                  }
                  frame #1 {
                    n542 = call "LoadDataSPC130.vi"("Path"=w583) -> ()  [unwired: 2 in, 3 out]
                  }
                  frame #2 {
                    n543 = call "LoadDataKen.vi"("Path"=w584) -> ()  [unwired: 5 in]
                  }
                }
              }
              frame #5 {
                n544 = stacked-sequence {
                  frame #0 {
                    n545 = call "TempRefnum.vi"("change?"=FALSE) -> ("refnum out"=w586:refnum<k1>)  [unwired: 1 in]
                    n546 = Close File(refnum=w586) -> (error out=w585:errorcluster)  [unwired: 1 in, 1 out]
                    n547 = call "HandleError.vi"("error in (no error)"=w585) -> ()
                  }
                  frame #1 {
                    n548 = call "TotalRecall_Reload.vi"() -> ("gap"=w588:i32, "invalid"=w589:i32, "valid"=w590:i32)  [unwired: 4 in, 1 out]
                    n549 = property on="total" class="DigNum (strict)"("Value"=w590) -> ()  [unwired: 2 in, 2 out]
                    n550 = property on="invalid" class="DigNum (strict)"("Value"=w589) -> ()  [unwired: 2 in, 2 out]
                    n551 = property on="gap" class="DigNum (strict)"("Value"=w588) -> ()  [unwired: 2 in, 2 out]
                  }
                  frame #2 {
                    n552 = call "sumofphotons.vi"("s"=FALSE) -> ("sum of photons out"=w592:u32[][][][])  [unwired: 1 in]
                    n553 = property on="plane" class="DigNum (strict)"() -> ("Value"=w595:u32)  [unwired: 2 in, 2 out]
                    n554 = property on="threshold" class="Clust (strict)"() -> ("Value"=w591:cluster{"max":u32, "min":u32})  [unwired: 2 in, 2 out]
                    n555 = property on="router" class="Ring (strict)"() -> ("Value"=w596:u8)  [unwired: 2 in, 2 out]
                    n556 = property on="RGB or false color?" class="Bool (strict)"() -> ("Value"=w597:bool)  [unwired: 2 in, 2 out]
                    n557 = call "OnlinePic.vi"("action"=T2."ini" ("Enum"), "RGB/False"=w597, "Threshold (max)"=w591, "plane"=w595, "router channel"=w596, "Array"=w592) -> ()  [unwired: 1 in, 5 out]
                  }
                  frame #3 {
                    n558 = call "ViewImageSetnew.vi"("action"=enum16{"Display", "change", "Get", "Set"}."Get" ("Enum")) -> ("Image Settings"=w601:T11)  [unwired: 2 in]
                    n559 = Unbundle By Name(w601) -> ("Image Size (pixel).z"=w600:u32)
                    n560 = case shown="0" w600 {
                      tunnel: [i8 2 w605] -> w599
                      tunnel: [u8 0 w605] -> w598
                      frame #0 {
                      }
                      frame #1 {
                        w605 = u8 0
                      }
                    }
                    n561 = property on="plane" class="DigNum (strict)"("Disabled"=w599, "Value"=w598) -> ()  [unwired: 2 in, 2 out]
                  }
                  frame #4 {
                    w606 = u8 0
                    n562 = property on="F2-Image" class="Boolean"("Disabled"=u8 0) -> ()  [unwired: 2 in, 2 out]
                    n563 = property on="Image LOADED" class="Boolean (strict)"("Blinking"=FALSE, "Value"=TRUE ("Image LOADED")) -> ()  [unwired: 2 in, 2 out]
                    n564 = property on="Lifetime pick" class="Boolean"("Disabled"=w606) -> ()  [unwired: 2 in, 2 out]
                    n565 = property on="RGB or false color?" class="Boolean (strict)"("Disabled"=w606) -> ()  [unwired: 2 in, 2 out]
                    n566 = property on="router" class="Ring (strict)"("Disabled"=w606) -> ()  [unwired: 2 in, 2 out]
                    n567 = property on="16bit" class="Boolean"("Disabled"=w606) -> ()  [unwired: 2 in, 2 out]
                    n568 = property on="threshold" class="Clust (strict)"("Disabled"=w606) -> ()  [unwired: 2 in, 2 out]
                    n569 = property on="coincidence spot" class="Boolean"("Disabled"=w606) -> ()  [unwired: 2 in, 2 out]
                    n570 = property on="TAC Window" class="Boolean"("Disabled"=w606) -> ()  [unwired: 2 in, 2 out]
                    n571 = property on="Export" class="Bool"("Disabled"=w606) -> ()  [unwired: 2 in, 2 out]
                    n572 = property on="coincidence\nimage" class="Bool"("Disabled"=w606) -> ()  [unwired: 2 in, 2 out]
                  }
                  frame #5 {
                    n573 = property on="Ampel" class="Clust (strict)"("Value"=cluster{"RED":bool, "RED 2":bool, "RED 3":bool} {"RED"=FALSE, "RED 2"=FALSE, "RED 3"=TRUE} ("Ampel")) -> ()  [unwired: 2 in, 2 out]
                  }
                }
              }
            }
          }
          event #17 {
            n574 = event-data() -> ("ItemTag"=w613:string)  [unwired: 1 in, 5 out]
            n575 = case shown="\"Spotfinder\"" w613 {
              tunnel: [_ _ TRUE _ _ _ _ _ _ _ _ _ _ _ _ _ _ _ _ _ _] -> w612
              frame #0 {
                n576 = control-ref of="Image Path"() -> (w614:refnum<vi>)
                n577 = property class="Path"(reference=w614) -> ("Value"=w615:path)  [unwired: 1 in, 2 out]
                n578 = Strip Path(path=w615) -> (stripped path=w616:path)  [unwired: 1 out]
                n579 = Not A Number/Path/Refnum?(number/path/refnum=w616) -> (NaN/Path/Refnum?=w617:bool)
                n580 = case shown="False" w617 {
                  tunnel: w616 -> [w620 _]
                  frame #0 {
                    n581 = call "fileformatGlobal.vi"() -> ("fileformat out"=w622:enum16{"Herty", "Ken", "SPC130", "HydraHarp"})  [unwired: 2 in]
                    n582 = case shown="\"SPC130\"" w622 {
                      tunnel: ["plane000line000.fifo" ("name or relative path") "plane000line000module000.spc" ("name or relative path") "0_0.ifif" ("name or relative path")] -> w621
                      frame #0 {
                      }
                      frame #1 {
                      }
                      frame #2 {
                      }
                    }
                    n583 = call "ViewFIFOSet.vi"("Enum"=enum16{"Display", "change", "Get", "Set"}."Get") -> ("FIFO Settings (Array)"=w628:T12[])  [unwired: 1 in]
                    n584 = Index Array(array=w628) -> (element=w618:T12)  [unwired: 1 in]
                    n585 = Unbundle By Name(w618) -> ("ADC.ADC Resolution"=w624:i32)
                    n586 = Not Equal To 0?(x=w624) -> (x != 0?=w623:bool)
                    n587 = Build Path(base path=w620, name or relative path=w621) -> (appended path=w619:path)
                    n588 = Select(t=enum16{"32 bit", "48 bit"}."48 bit" ("File Type"), s=w623, f=enum16{"32 bit", "48 bit"}."32 bit" ("File Type")) -> (s? t:f=w627:enum16{"32 bit", "48 bit"})
                    n589 = call "FIFORawDataScreener.vi"("File Type"=w627, "Path"=w619) -> ()  [unwired: 2 in]
                  }
                  frame #1 {
                    n590 = One Button Dialog(message="Select header file first!") -> ()  [unwired: 1 in, 1 out]
                  }
                }
              }
              frame #1 {
                n591 = call "ViewFIFOTrace.vi"() -> ()  [unwired: 1 in]
              }
              frame #2 {
              }
              frame #3 {
                n592 = stacked-sequence {
                  seq-local: [_ _ _ _ w668 _] -> [_ _ _ _ _ w680]
                  frame #0 {
                    n593 = control-ref of="notes"() -> (w639:refnum<vi>)
                    n594 = property class="Str"(reference=w639) -> (reference out=w635:refnum<vi>, "Value"=w637:string)  [unwired: 1 in, 1 out]
                    n595 = Not Equal?(x=w637, y="") -> (x != y?=w636:bool)
                    n596 = case shown="True" w636 {
                      tunnel: w635 -> [_ w640]
                      frame #0 {
                      }
                      frame #1 {
                        n597 = call "SaveNotes.vi"("Enum"=enum16{"Get Path", "Read", "Save"}."Save", "String"=w640) -> ()  [unwired: 3 in]
                      }
                    }
                  }
                  frame #1 {
                    w656 = FALSE ("Boolean")
                    w649 = u8 2 ("Disabled")
                    n598 = property on="TACwinLoaded?" class="Boolean (strict)"("Value"=FALSE ("TACwinLoaded?")) -> ()  [unwired: 2 in, 2 out]
                    n599 = property on="F2-Image" class="Boolean"("Disabled"=u8 2) -> ()  [unwired: 2 in, 2 out]
                    n600 = property on="TAC Window" class="Boolean"("Disabled"=2) -> ()  [unwired: 2 in, 2 out]
                    n601 = property on="LOADED HDR" class="Bool (strict)"("Value"=w656) -> ()  [unwired: 2 in, 2 out]
                    n602 = property on="Image LOADED" class="Boolean (strict)"("Value"=w656, "Blinking"=FALSE) -> ()  [unwired: 2 in, 2 out]
                    n603 = property on="Image Path" class="Path"("Disabled"=u8 0) -> ()  [unwired: 2 in, 2 out]
                    n604 = property on="Load" class="Bool"("Visible"=TRUE) -> ()  [unwired: 2 in, 2 out]
                    n605 = property on="RGB or false color?" class="Boolean (strict)"("Disabled"=w649, "Value"=w656) -> ()  [unwired: 2 in, 2 out]
                    n606 = property on="Lifetime pick" class="Boolean"("Disabled"=w649) -> ()  [unwired: 2 in, 2 out]
                    n607 = property on="router" class="Ring (strict)"("Disabled"=w649) -> ()  [unwired: 2 in, 2 out]
                    n608 = property on="plane" class="DigNum (strict)"("Disabled"=w649) -> ()  [unwired: 2 in, 2 out]
                    n609 = property on="Export" class="Boolean"("Disabled"=w649) -> ()  [unwired: 2 in, 2 out]
                    n610 = property on="View Image Settings" class="Boolean"("Disabled"=w649) -> ()  [unwired: 2 in, 2 out]
                    n611 = property on="View FIFO Settings" class="Boolean"("Disabled"=w649) -> ()  [unwired: 2 in, 2 out]
                    n612 = property on="Load Image" class="Boolean"("Disabled"=w649, "Visible"=FALSE) -> ()  [unwired: 2 in, 2 out]
                    n613 = property on="16bit" class="Boolean"("Disabled"=w649) -> ()  [unwired: 2 in, 2 out]
                    n614 = property on="Spotfinder" class="Boolean"("Disabled"=w649) -> ()  [unwired: 2 in, 2 out]
                    n615 = property on="notes" class="String"("Value"="") -> ()  [unwired: 2 in, 2 out]
                    n616 = property on="invalid" class="DigNum (strict)"("Value"=u32 0 ("invalid photons")) -> ()  [unwired: 2 in, 2 out]
                    n617 = property on="gap" class="DigNum (strict)"("Value"=u32 0 ("gap photons")) -> ()  [unwired: 2 in, 2 out]
                    n618 = property on="total" class="DigNum (strict)"("Value"=u32 0 ("invalid photons")) -> ()  [unwired: 2 in, 2 out]
                    n619 = call "sumofphotons.vi"("s"=TRUE, "sum of photons"=u32[][][][] []) -> ()  [unwired: 1 out]
                  }
                  frame #2 {
                    n620 = call "IMAQ WindClose"("Close All Windows (False)"=TRUE ("Close All Windows (N)")) -> ("error out"=w663:errorcluster)  [unwired: 5 in]
                    n621 = call "IMAQ Dispose"("All Images? (No)"=TRUE, "error in (no error)"=w663) -> ("error out"=w664:errorcluster)  [unwired: 4 in]
                    n622 = call "IMAQ WindToolsClose"("error in (no error)"=w664) -> ("error out"=w657:errorcluster)  [unwired: 5 in]
                    n623 = call "Intensityduplex.vi"("Enum"=T3."dump") -> ()  [unwired: 4 in, 2 out]
                    n624 = call "OnlinePic.vi"("action"=T2."clear" ("Enum")) -> ()  [unwired: 6 in, 5 out]
                    n625 = call "16bitImageglobal.vi"("Enum"=T4."Ini") -> ()  [unwired: 4 in, 4 out]
                    n626 = call "HandleError.vi"("error in (no error)"=w657) -> ()
                    n627 = Wait Until Next ms Multiple(millisecond multiple=u32 2500) -> ()  [unwired: 1 out]
                  }
                  frame #3 {
                    n628 = property on="Ampel" class="Clust (strict)"("Value"=cluster{"RED":bool, "RED 2":bool, "RED 3":bool} {"RED"=TRUE, "RED 2"=FALSE, "RED 3"=FALSE} ("Ampel")) -> ()  [unwired: 2 in, 2 out]
                  }
                  frame #4 {
                    (unwired) T10."existing file" ("select mode (2)")
                    n629 = File Dialog(6:"*.hdr; fileinfo.txt" ("pattern"), 7:"Select header file ... (quick view)" ("prompt")) -> (0:w667:errorcluster, 1:w669:bool, 3:w670:path)  [unwired: 5 in, 1 out]
                    n630 = Unbundle(w667) -> ()  [unwired: 3 out]
                    n631 = case shown="False" w669 {
                      tunnel: w670 -> [w675 _]
                      tunnel: [1 0] -> w668
                      frame #0 {
                        n632 = control-ref of="Image Path"() -> (w674:refnum<vi>)
                        n633 = call "LoadHeaderKenandHerty.vi"("appended path"=w675, "reference"=w674) -> ()  [unwired: 3 in, 1 out]
                        n634 = Path To String(path=w675) -> (string=w676:string)
                        n635 = Concatenate Strings("Anna_linescan " ("string"), w676) -> (w678:string)
                        n636 = property class="VI"("Front Panel Window:Title"=w678) -> ()  [unwired: 2 in, 2 out]
                      }
                      frame #1 {
                      }
                    }
                  }
                  frame #5 {
                    n637 = for {
                      N: w680 -> [_]
                      n638 = stacked-sequence {
                        frame #0 {
                          w681 = u8 0 ("Disabled")
                          n639 = property on="LOADED HDR" class="Bool (strict)"("Value"=TRUE ("Boolean")) -> ()  [unwired: 2 in, 2 out]
                          n640 = property on="Load" class="Bool"("Visible"=FALSE) -> ()  [unwired: 2 in, 2 out]
                          n641 = property on="Image LOADED" class="Boolean (strict)"("Disabled"=w681) -> ()  [unwired: 2 in, 2 out]
                          n642 = property on="View Image Settings" class="Boolean"("Disabled"=w681) -> ()  [unwired: 2 in, 2 out]
                          n643 = property on="View FIFO Settings" class="Boolean"("Disabled"=w681) -> ()  [unwired: 2 in, 2 out]
                          n644 = control-ref of="notes"() -> (w687:refnum<vi>)
                          n645 = control-ref of="Image Path"() -> (w685:refnum<vi>)
                          n646 = property on="Ampel" class="Clust (strict)"("Value"=cluster{"RED":bool, "RED 2":bool, "RED 3":bool} {"RED"=TRUE, "RED 2"=TRUE, "RED 3"=FALSE} ("Ampel")) -> ()  [unwired: 2 in, 2 out]
                          n647 = call "SaveNotes.vi"("Enum"=enum16{"Get Path", "Read", "Save"}."Get Path", "String"=w687, "Path"=w685) -> ()  [unwired: 2 in]
                        }
                        frame #1 {
                          n648 = call "ViewImageSetnew.vi"("action"=enum16{"Display", "change", "Get", "Set"}."Get" ("Enum")) -> ("Image Settings"=w689:T11)  [unwired: 2 in]
                          n649 = Unbundle By Name(w689) -> ("Retrace"=w688:bool)
                          n650 = case shown="False" w688 {
                            frame #0 {
                              n651 = property on="Load Image" class="Boolean"("Disabled"=u8 0, "Visible"=TRUE) -> ()  [unwired: 2 in, 2 out]
                            }
                            frame #1 {
                              n652 = property on="Load Image" class="Boolean"("Disabled"=u8 2, "Visible"=FALSE) -> ()  [unwired: 2 in, 2 out]
                              n653 = One Button Dialog(message="Die Retrace kann derzeit noch nicht bearbeitet werden.") -> ()  [unwired: 1 in, 1 out]
                            }
                          }
                        }
                        frame #2 {
                          n654 = property on="Image Path" class="Path"("Disabled"=u8 2) -> ()  [unwired: 2 in, 2 out]
                          n655 = property on="Load Image" class="Boolean"("Disabled"=u8 2) -> ()  [unwired: 2 in, 2 out]
                          n656 = property on="Image LOADED" class="Boolean (strict)"("Blinking"=TRUE) -> ()  [unwired: 2 in, 2 out]
                          n657 = call "sumofphotons.vi"("s"=TRUE, "sum of photons"=u32[][][][] []) -> ()  [unwired: 1 out]
                        }
                        frame #3 {
                          n658 = control-ref of="Image Path"() -> (w705:refnum<vi>)
                          n659 = call "fileformatGlobal.vi"() -> ("fileformat out"=w704:enum16{"Herty", "Ken", "SPC130", "HydraHarp"})  [unwired: 2 in]
                          n660 = call "QuickLoadData.vi"("Fileformat"=w704, "Path"=w705) -> ("gap photons"=w701:u32, "invalid photons"=w703:u32, "total"=w702:u32)  [unwired: 1 in]
                          n661 = property on="invalid" class="DigNum (strict)"("Value"=w702) -> ()  [unwired: 2 in, 2 out]
                          n662 = property on="total" class="DigNum (strict)"("Value"=w703) -> ()  [unwired: 2 in, 2 out]
                          n663 = property on="gap" class="DigNum (strict)"("Value"=w701) -> ()  [unwired: 2 in, 2 out]
                        }
                        frame #4 {
                          n664 = call "sumofphotons.vi"("s"=FALSE) -> ("sum of photons out"=w708:u32[][][][])  [unwired: 1 in]
                          n665 = property on="threshold" class="Clust (strict)"() -> ("Value"=w706:cluster{"max":u32, "min":u32})  [unwired: 2 in, 2 out]
                          n666 = property on="router" class="Ring (strict)"() -> ("Value"=w711:u8)  [unwired: 2 in, 2 out]
                          n667 = property on="plane" class="DigNum (strict)"() -> ("Value"=w712:u32)  [unwired: 2 in, 2 out]
                          n668 = property on="RGB or false color?" class="Bool (strict)"() -> ("Value"=w710:bool)  [unwired: 2 in, 2 out]
                          n669 = call "OnlinePic.vi"("action"=T2."ini" ("Enum"), "RGB/False"=w710, "Threshold (max)"=w706, "plane"=w712, "router channel"=w711, "Array"=w708) -> ()  [unwired: 1 in, 5 out]
                        }
                        frame #5 {
                          n670 = call "ViewImageSetnew.vi"("action"=enum16{"Display", "change", "Get", "Set"}."Get" ("Enum")) -> ("Image Settings"=w714:T11)  [unwired: 2 in]
                          n671 = Unbundle By Name(w714) -> ("Image Size (pixel).z"=w715:u32)
                          n672 = case shown="0" w715 {
                            tunnel: [i8 2 w720] -> w716
                            tunnel: [u8 0 w720] -> w717
                            frame #0 {
                            }
                            frame #1 {
                              w720 = u8 0
                            }
                          }
                          n673 = property on="plane" class="DigNum (strict)"("Disabled"=w716, "Value"=w717) -> ()  [unwired: 2 in, 2 out]
                        }
                        frame #6 {
                          w721 = u8 0
                          w722 = u8 2 ("Disabled")
                          n674 = property on="Image LOADED" class="Boolean (strict)"("Blinking"=FALSE, "Value"=TRUE ("Image LOADED")) -> ()  [unwired: 2 in, 2 out]
                          n675 = property on="Lifetime pick" class="Boolean"("Disabled"=w722) -> ()  [unwired: 2 in, 2 out]
                          n676 = property on="TAC Window" class="Boolean"("Disabled"=w722) -> ()  [unwired: 2 in, 2 out]
                          n677 = property on="coincidence spot" class="Boolean"("Disabled"=w722) -> ()  [unwired: 2 in, 2 out]
                          n678 = property on="coincidence\nimage" class="Bool"("Disabled"=w722) -> ()  [unwired: 2 in, 2 out]
                          n679 = property on="RGB or false color?" class="Boolean (strict)"("Disabled"=w721) -> ()  [unwired: 2 in, 2 out]
                          n680 = property on="router" class="Ring (strict)"("Disabled"=w721) -> ()  [unwired: 2 in, 2 out]
                          n681 = property on="16bit" class="Boolean"("Disabled"=w721) -> ()  [unwired: 2 in, 2 out]
                          n682 = property on="Export" class="Bool"("Disabled"=w721) -> ()  [unwired: 2 in, 2 out]
                          n683 = property on="threshold" class="Clust (strict)"("Disabled"=w721) -> ()  [unwired: 2 in, 2 out]
                        }
                        frame #7 {
                          n684 = property on="Ampel" class="Clust (strict)"("Value"=cluster{"RED":bool, "RED 2":bool, "RED 3":bool} {"RED"=FALSE, "RED 2"=FALSE, "RED 3"=TRUE} ("Ampel")) -> ()  [unwired: 2 in, 2 out]
                        }
                      }
                    }
                  }
                }
              }
              frame #4 {
                n685 = stacked-sequence {
                  seq-local: [_ w739 _] -> [_ _ w751]
                  frame #0 {
                    n686 = property on="LOADED HDR" class="Boolean (strict)"() -> ("Value"=w733:bool)  [unwired: 2 in, 2 out]
                    n687 = case shown="True" w733 {
                      frame #0 {
                      }
                      frame #1 {
                        w737 = FALSE ("Boolean")
                        w736 = u8 2 ("Disabled")
                        n688 = property on="Image LOADED" class="Boolean (strict)"("Value"=w737, "Blinking"=w737) -> ()  [unwired: 2 in, 2 out]
                        n689 = property on="Spotfinder" class="Boolean"("Disabled"=w736) -> ()  [unwired: 2 in, 2 out]
                        n690 = property on="TAC Window" class="Boolean"("Disabled"=w736) -> ()  [unwired: 2 in, 2 out]
                        n691 = property on="Export" class="Boolean"("Disabled"=w736) -> ()  [unwired: 2 in, 2 out]
                        n692 = property on="View Image Settings" class="Boolean"("Disabled"=w736) -> ()  [unwired: 2 in, 2 out]
                        n693 = property on="View FIFO Settings" class="Boolean"("Disabled"=w736) -> ()  [unwired: 2 in, 2 out]
                      }
                    }
                    n694 = control-ref of="notes"() -> (w726:refnum<vi>)
                    n695 = property class="Str"(reference=w726) -> (reference out=w727:refnum<vi>, "Value"=w729:string)  [unwired: 1 in, 1 out]
                    n696 = Not Equal?(x=w729, y="") -> (x != y?=w728:bool)
                    n697 = case shown="True" w728 {
                      tunnel: w727 -> [_ w734]
                      frame #0 {
                      }
                      frame #1 {
                        n698 = call "SaveNotes.vi"("Enum"=enum16{"Get Path", "Read", "Save"}."Save", "String"=w734) -> ()  [unwired: 3 in]
                      }
                    }
                    n699 = call "Intensityduplex.vi"("Enum"=T3."dump") -> ()  [unwired: 4 in, 2 out]
                    n700 = call "OnlinePic.vi"("action"=T2."clear" ("Enum")) -> ()  [unwired: 6 in, 5 out]
                  }
                  frame #1 {
                    (unwired) T10."existing file" ("select mode (2)")
                    n701 = File Dialog(6:"*.hdr; fileinfo.txt" ("pattern"), 7:"Select header file ..." ("prompt")) -> (0:w738:errorcluster, 1:w743:bool, 3:w742:path)  [unwired: 5 in, 1 out]
                    n702 = Unbundle(w738) -> ()  [unwired: 3 out]
                    n703 = case shown="False" w743 {
                      tunnel: w742 -> [w745 _]
                      tunnel: [1 0] -> w739
                      frame #0 {
                        n704 = control-ref of="Image Path"() -> (w746:refnum<vi>)
                        n705 = Path To String(path=w745) -> (string=w747:string)
                        n706 = call "LoadHeaderKenandHerty.vi"("appended path"=w745, "reference"=w746) -> ()  [unwired: 3 in, 1 out]
                        n707 = Concatenate Strings("Anna_linescan " ("string"), w747) -> (w749:string)
                        n708 = property class="VI"("Front Panel Window:Title"=w749) -> ()  [unwired: 2 in, 2 out]
                      }
                      frame #1 {
                      }
                    }
                  }
                  frame #2 {
                    n709 = for {
                      N: w751 -> [_]
                      n710 = stacked-sequence {
                        frame #0 {
                          w759 = u8 0 ("Disabled")
                          n711 = property on="Image LOADED" class="Boolean (strict)"("Disabled"=w759) -> ()  [unwired: 2 in, 2 out]
                          n712 = property on="View Image Settings" class="Boolean"("Disabled"=w759) -> ()  [unwired: 2 in, 2 out]
                          n713 = property on="View FIFO Settings" class="Boolean"("Disabled"=w759) -> ()  [unwired: 2 in, 2 out]
                          n714 = property on="LOADED HDR" class="Bool (strict)"("Value"=TRUE ("Boolean")) -> ()  [unwired: 2 in, 2 out]
                          n715 = control-ref of="notes"() -> (w752:refnum<vi>)
                          n716 = control-ref of="Image Path"() -> (w754:refnum<vi>)
                          n717 = property on="Ampel" class="Clust (strict)"("Value"=cluster{"RED":bool, "RED 2":bool, "RED 3":bool} {"RED"=TRUE, "RED 2"=TRUE, "RED 3"=FALSE} ("Ampel")) -> ()  [unwired: 2 in, 2 out]
                          n718 = call "SaveNotes.vi"("Enum"=enum16{"Get Path", "Read", "Save"}."Get Path", "String"=w752, "Path"=w754) -> ()  [unwired: 2 in]
                          n719 = call "ViewImageSetnew.vi"("action"=enum16{"Display", "change", "Get", "Set"}."Get" ("Enum")) -> ("Image Settings"=w756:T11)  [unwired: 2 in]
                          n720 = Unbundle By Name(w756) -> ("Retrace"=w757:bool)
                          n721 = property on="Load" class="Bool"("Visible"=FALSE) -> ()  [unwired: 2 in, 2 out]
                          n722 = case shown="False" w757 {
                            frame #0 {
                              n723 = property on="Load Image" class="Boolean"("Disabled"=u8 0, "Visible"=TRUE) -> ()  [unwired: 2 in, 2 out]
                            }
                            frame #1 {
                              n724 = property on="Load Image" class="Boolean"("Disabled"=u8 2, "Visible"=FALSE) -> ()  [unwired: 2 in, 2 out]
                              n725 = One Button Dialog(message="Die Retrace kann derzeit noch nicht bearbeitet werden.") -> ()  [unwired: 1 in, 1 out]
                            }
                          }
                        }
                        frame #1 {
                          n726 = property on="Image LOADED" class="Boolean (strict)"("Blinking"=TRUE) -> ()  [unwired: 2 in, 2 out]
                          n727 = property on="Image Path" class="Path"("Disabled"=u8 2) -> ()  [unwired: 2 in, 2 out]
                          n728 = property on="Load Image" class="Boolean"("Disabled"=u8 2) -> ()  [unwired: 2 in, 2 out]
                          n729 = call "sumofphotons.vi"("s"=TRUE, "sum of photons"=u32[][][][] []) -> ()  [unwired: 1 out]
                        }
                        frame #2 {
                          n730 = call "TempPath.vi"("change"=FALSE) -> ("stripped path 2"=w775:path)  [unwired: 2 in]
                          n731 = Build Path(base path=w775, name or relative path="Anna_linescan.tmp" ("prompt")) -> (appended path=w777:path)
                          n732 = call <vilib>:"compatOverwrite.vi"("overwrite (F)"=TRUE) -> ("overwrite?"=w772:T14)
                          n733 = Open/Create/Replace Datalog(5:T8 {"router"=[], "macro times"=[], "micro times"=[], "invalid"=[], "gap"=[]} ("cluster"), 10:w772, 11:w777) -> (3:w780:refnum<k1>)  [unwired: 3 in, 2 out]
                          n734 = call "TempRefnum.vi"("change?"=TRUE, "refnum in"=w780) -> ()  [unwired: 1 out]
                        }
                        frame #3 {
                          n735 = property on="LOADED HDR" class="Bool (strict)"() -> ("Value"=w781:bool)  [unwired: 2 in, 2 out]
                          n736 = case shown="True" w781 {
                            frame #0 {
                            }
                            frame #1 {
                              n737 = control-ref of="Image Path"() -> (w783:refnum<vi>)
                              n738 = call "fileformatGlobal.vi"() -> ("fileformat out"=w782:enum16{"Herty", "Ken", "SPC130", "HydraHarp"})  [unwired: 2 in]
                              n739 = case shown="\"Ken\"" w782 {
                                tunnel: w783 -> [w784 w785 w786]
                                frame #0 {
                                n740 = call "LoadDataSPC130.vi"("Path"=w784) -> ()  [unwired: 2 in, 3 out]
                                }
                                frame #1 {
                                n741 = call "LoadData.vi"("Path"=w785) -> ()  [unwired: 2 in, 3 out]
                                }
                                frame #2 {
                                n742 = call "LoadDataKen.vi"("Path"=w786) -> ()  [unwired: 5 in]
                                }
                              }
                            }
                          }
                        }
                        frame #4 {
                          n743 = call "TempRefnum.vi"("change?"=FALSE) -> ("refnum out"=w788:refnum<k1>)  [unwired: 1 in]
                          n744 = Close File(refnum=w788) -> (error out=w787:errorcluster)  [unwired: 1 in, 1 out]
                          n745 = call "HandleError.vi"("error in (no error)"=w787) -> ()
                        }
                        frame #5 {
                          n746 = call "TotalRecall_Reload.vi"() -> ("gap"=w790:i32, "invalid"=w791:i32, "valid"=w792:i32)  [unwired: 4 in, 1 out]
                          n747 = property on="total" class="DigNum (strict)"("Value"=w792) -> ()  [unwired: 2 in, 2 out]
                          n748 = property on="invalid" class="DigNum (strict)"("Value"=w791) -> ()  [unwired: 2 in, 2 out]
                          n749 = property on="gap" class="DigNum (strict)"("Value"=w790) -> ()  [unwired: 2 in, 2 out]
                        }
                        frame #6 {
                          n750 = call "sumofphotons.vi"("s"=FALSE) -> ("sum of photons out"=w794:u32[][][][])  [unwired: 1 in]
                          n751 = property on="router" class="Ring (strict)"() -> ("Value"=w798:u8)  [unwired: 2 in, 2 out]
                          n752 = property on="plane" class="DigNum (strict)"() -> ("Value"=w797:u32)  [unwired: 2 in, 2 out]
                          n753 = property on="threshold" class="Clust (strict)"() -> ("Value"=w793:cluster{"max":u32, "min":u32})  [unwired: 2 in, 2 out]
                          n754 = property on="RGB or false color?" class="Bool (strict)"() -> ("Value"=w799:bool)  [unwired: 2 in, 2 out]
                          n755 = call "OnlinePic.vi"("action"=T2."ini" ("Enum"), "RGB/False"=w799, "Threshold (max)"=w793, "plane"=w797, "router channel"=w798, "Array"=w794) -> ()  [unwired: 1 in, 5 out]
                        }
                        frame #7 {
                          n756 = call "ViewImageSetnew.vi"("action"=enum16{"Display", "change", "Get", "Set"}."Get" ("Enum")) -> ("Image Settings"=w801:T11)  [unwired: 2 in]
                          n757 = Unbundle By Name(w801) -> ("Image Size (pixel).z"=w802:u32)
                          n758 = case shown="0" w802 {
                            tunnel: [i8 2 w807] -> w803
                            tunnel: [u8 0 w807] -> w804
                            frame #0 {
                            }
                            frame #1 {
                              w807 = u8 0
                            }
                          }
                          n759 = property on="plane" class="DigNum (strict)"("Disabled"=w803, "Value"=w804) -> ()  [unwired: 2 in, 2 out]
                        }
                        frame #8 {
                          w809 = u8 0 ("Disabled")
                          w808 = u8 0
                          n760 = property on="Image LOADED" class="Boolean (strict)"("Blinking"=FALSE, "Value"=TRUE ("Image LOADED")) -> ()  [unwired: 2 in, 2 out]
                          n761 = property on="Lifetime pick" class="Boolean"("Disabled"=w808) -> ()  [unwired: 2 in, 2 out]
                          n762 = property on="RGB or false color?" class="Boolean (strict)"("Disabled"=w808) -> ()  [unwired: 2 in, 2 out]
                          n763 = property on="router" class="Ring (strict)"("Disabled"=w808) -> ()  [unwired: 2 in, 2 out]
                          n764 = property on="16bit" class="Boolean"("Disabled"=w808) -> ()  [unwired: 2 in, 2 out]
                          n765 = property on="threshold" class="Clust (strict)"("Disabled"=w808) -> ()  [unwired: 2 in, 2 out]
                          n766 = property on="coincidence spot" class="Boolean"("Disabled"=w808) -> ()  [unwired: 2 in, 2 out]
                          n767 = property on="F2-Image" class="Boolean"("Disabled"=w809) -> ()  [unwired: 2 in, 2 out]
                          n768 = property on="TAC Window" class="Boolean"("Disabled"=w808) -> ()  [unwired: 2 in, 2 out]
                          n769 = property on="Export" class="Bool"("Disabled"=w808) -> ()  [unwired: 2 in, 2 out]
                          n770 = property on="Spotfinder" class="Boolean"("Disabled"=w809) -> ()  [unwired: 2 in, 2 out]
                          n771 = property on="coincidence\nimage" class="Bool"("Disabled"=w808) -> ()  [unwired: 2 in, 2 out]
                        }
                        frame #9 {
                          n772 = property on="Ampel" class="Clust (strict)"("Value"=cluster{"RED":bool, "RED 2":bool, "RED 3":bool} {"RED"=FALSE, "RED 2"=FALSE, "RED 3"=TRUE} ("Ampel")) -> ()  [unwired: 2 in, 2 out]
                        }
                      }
                    }
                  }
                }
              }
              frame #5 {
                n773 = property on="Image Path" class="Path"() -> ("Value"=w813:path)  [unwired: 2 in, 2 out]
                n774 = call "imagemanipulation.vi"("Results"=w813) -> ()  [unwired: 7 in]
              }
              frame #6 {
                n775 = stacked-sequence {
                  frame #0 {
                    n776 = property on="Ampel" class="Clust (strict)"("Value"=cluster{"RED":bool, "YELLOW":bool, "GREEN":bool} {"RED"=FALSE, "YELLOW"=FALSE, "GREEN"=FALSE} ("Ampel")) -> ("Controls[]"=w815:refnum<vi>[])  [unwired: 2 in, 2 out]
                    n777 = Index Array(array=w815, index=1) -> (element=w817:refnum<vi>)
                    n778 = property class="Ctl"(reference=w817, "Blinking"=TRUE) -> ()  [unwired: 1 in, 2 out]
                  }
                  frame #1 {
                    n779 = control-ref of="notes"() -> ()  [unwired: 1 out]
                  }
                  frame #2 {
                    n780 = property on="Ampel" class="Clust (strict)"("Value"=cluster{"RED":bool, "YELLOW":bool, "GREEN":bool} {"RED"=FALSE, "YELLOW"=FALSE, "GREEN"=TRUE} ("Ampel")) -> ("Controls[]"=w822:refnum<vi>[])  [unwired: 2 in, 2 out]
                    n781 = Index Array(array=w822, index=1) -> (element=w820:refnum<vi>)
                    n782 = property class="Ctl"(reference=w820, "Blinking"=FALSE) -> ()  [unwired: 1 in, 2 out]
                  }
                }
              }
              frame #7 {
                n783 = control-ref of="Image Path"() -> (w824:refnum<vi>)
                n784 = control-ref of="notes"() -> (w825:refnum<vi>)
                n785 = call "TimeGatedImage.vi"("Image Path"=w824, "notes 3"=w825) -> ()  [unwired: 2 in]
              }
              frame #8 {
                n786 = call "Splashscreen.vi"("Mode"=enum16{"splash", "dialog"}."dialog") -> ()  [unwired: 1 in]
              }
              frame #9 {
                n787 = call "ViewFIFOSet.vi"("Enum"=enum16{"Display", "change", "Get", "Set"}."Display") -> ()  [unwired: 1 in, 1 out]
              }
              frame #10 {
                n788 = call "ViewImageSetnew.vi"("action"=enum16{"Display", "change", "Get", "Set"}."Display" ("Enum")) -> ()  [unwired: 2 in, 1 out]
              }
              frame #11 {
                n789 = control-ref of="Image Path"() -> (w829:refnum<vi>)
                n790 = call "GetSetTempDir.vi"("Path"=w829) -> ()  [unwired: 4 in]
              }
              frame #12 {
                n791 = control-ref of="Int duplex?"() -> (w834:refnum<vi>)
                n792 = control-ref of="16btimage?"() -> (w833:refnum<vi>)
                n793 = control-ref of="does a coinc image exist?"() -> (w832:refnum<vi>)
                n794 = control-ref of="Image Path"() -> (w830:refnum<vi>)
                n795 = control-ref of="notes"() -> (w831:refnum<vi>)
                n796 = call "ExportDialog.vi"("Int duplex ctl"=w834, "16 bit ctl"=w833, "coincidence image ctl"=w832, "Path"=w830, "notes 2"=w831) -> ()  [unwired: 4 in]
              }
              frame #13 {
                n797 = while {
                  stop <- w835 stop-if-true
                  n798 = property on="Image LOADED" class="Bool (strict)"() -> ("Value"=w835:bool)  [unwired: 2 in, 2 out]
                  n799 = case shown="True" w835 {
                    frame #0 {
                      n800 = while {
                        shift-right: [w838] -> _
                        shift-left: 9 -> [w839]
                        stop <- w837 stop-if-true
                        n801 = case shown="4" w839 {
                          tunnel: [1 2 3 4 10 6 7 8 _ _ _] -> w838
                          tunnel: [w845 _ _ _ _ _ _ _ _ _ _] -> w837
                          frame #0 {
                            n802 = while {
                              tunnel: [w852] -> w840
                              tunnel: [w848] -> w845
                              stop <- w849 continue-if-true
                              (unwired) T10."existing file" ("select mode (2)")
                              n803 = File Dialog(6:"*.hdr; fileinfo.txt" ("pattern"), 7:"Select header file" ("prompt")) -> (0:w847:errorcluster, 1:w848:bool, 3:w852:path)  [unwired: 5 in, 1 out]
                              n804 = Unbundle(w847) -> ()  [unwired: 3 out]
                              n805 = Not(x=w848) -> (.not. x?=w851:bool)
                              n806 = Not A Number/Path/Refnum?(number/path/refnum=w852) -> (NaN/Path/Refnum?=w850:bool)
                              n807 = And(x=w851, y=w850) -> (x .and. y?=w849:bool)
                            }
                            n808 = control-ref of="Image Path"() -> (w844:refnum<vi>)
                            n809 = Path To String(path=w840) -> (string=w843:string)
                            n810 = call "LoadHeaderKenandHerty.vi"("appended path"=w840, "reference"=w844) -> ()  [unwired: 3 in, 1 out]
                            n811 = Concatenate Strings("Anna_linescan " ("string"), w843) -> (w841:string)
                            n812 = property class="VI"("Front Panel Window:Title"=w841) -> ()  [unwired: 2 in, 2 out]
                          }
                          frame #1 {
                            w856 = u8 0 ("Disabled")
                            n813 = property on="Load" class="Bool"("Visible"=FALSE) -> ()  [unwired: 2 in, 2 out]
                            n814 = property on="LOADED HDR" class="Bool (strict)"("Value"=TRUE ("Boolean")) -> ()  [unwired: 2 in, 2 out]
                            n815 = property on="Image LOADED" class="Boolean (strict)"("Disabled"=w856) -> ()  [unwired: 2 in, 2 out]
                            n816 = property on="View Image Settings" class="Boolean"("Disabled"=w856) -> ()  [unwired: 2 in, 2 out]
                            n817 = property on="View FIFO Settings" class="Boolean"("Disabled"=w856) -> ()  [unwired: 2 in, 2 out]
                            n818 = property on="Ampel" class="Clust (strict)"("Value"=cluster{"RED":bool, "RED 2":bool, "RED 3":bool} {"RED"=TRUE, "RED 2"=TRUE, "RED 3"=FALSE} ("Ampel")) -> ()  [unwired: 2 in, 2 out]
                            n819 = call "ViewImageSetnew.vi"("action"=enum16{"Display", "change", "Get", "Set"}."Get" ("Enum")) -> ("Image Settings"=w864:T11)  [unwired: 2 in]
                            n820 = control-ref of="notes"() -> (w862:refnum<vi>)
                            n821 = control-ref of="Image Path"() -> (w860:refnum<vi>)
                            n822 = Unbundle By Name(w864) -> ("Retrace"=w863:bool)
                            n823 = call "SaveNotes.vi"("Enum"=enum16{"Get Path", "Read", "Save"}."Get Path", "String"=w862, "Path"=w860) -> ()  [unwired: 2 in]
                            n824 = case shown="False" w863 {
                              frame #0 {
                                n825 = property on="Load Image" class="Boolean"("Disabled"=u8 0, "Visible"=TRUE) -> ()  [unwired: 2 in, 2 out]
                              }
                              frame #1 {
                                n826 = property on="Load Image" class="Boolean"("Disabled"=u8 2, "Visible"=FALSE) -> ()  [unwired: 2 in, 2 out]
                                n827 = One Button Dialog(message="Die Retrace kann derzeit noch nicht bearbeitet werden.") -> ()  [unwired: 1 in, 1 out]
                              }
                            }
                          }
                          frame #2 {
                            n828 = property on="Image LOADED" class="Boolean (strict)"("Blinking"=TRUE) -> ()  [unwired: 2 in, 2 out]
                            n829 = property on="Image Path" class="Path"("Disabled"=u8 2) -> ()  [unwired: 2 in, 2 out]
                            n830 = property on="Load Image" class="Boolean"("Disabled"=u8 2) -> ()  [unwired: 2 in, 2 out]
                            n831 = call "sumofphotons.vi"("s"=TRUE, "sum of photons"=u32[][][][] []) -> ()  [unwired: 1 out]
                          }
                          frame #3 {
                            n832 = call "TempPath.vi"("change"=FALSE) -> ("stripped path 2"=w884:path)  [unwired: 2 in]
                            n833 = Build Path(base path=w884, name or relative path="Anna_linescan.tmp" ("prompt")) -> (appended path=w882:path)
                            n834 = call <vilib>:"compatOverwrite.vi"("overwrite (F)"=TRUE) -> ("overwrite?"=w877:T14)
                            n835 = Open/Create/Replace Datalog(5:T8 {"router"=[], "macro times"=[], "micro times"=[], "invalid"=[], "gap"=[]} ("cluster"), 10:w877, 11:w882) -> (3:w880:refnum<k1>)  [unwired: 3 in, 2 out]
                            n836 = call "TempRefnum.vi"("change?"=TRUE, "refnum in"=w880) -> ()  [unwired: 1 out]
                          }
                          frame #4 {
                            n837 = property on="LOADED HDR" class="Bool (strict)"() -> ("Value"=w888:bool)  [unwired: 2 in, 2 out]
                            n838 = case shown="True" w888 {
                              frame #0 {
                              }
                              frame #1 {
                                n839 = control-ref of="Image Path"() -> (w890:refnum<vi>)
                                n840 = call "fileformatGlobal.vi"() -> ("fileformat out"=w889:enum16{"Herty", "Ken", "SPC130", "HydraHarp"})  [unwired: 2 in]
                                n841 = case shown="\"SPC130\"" w889 {
                                tunnel: w890 -> [w891 w892 w893]
                                frame #0 {
                                n842 = call "LoadData.vi"("Path"=w891) -> ()  [unwired: 2 in, 3 out]
                                }
                                frame #1 {
                                n843 = call "LoadDataSPC130.vi"("Path"=w892) -> ()  [unwired: 2 in, 3 out]
                                }
                                frame #2 {
                                n844 = call "LoadDataKen.vi"("Path"=w893) -> ()  [unwired: 5 in]
                                }
                                }
                              }
                            }
                          }
                          frame #5 {
                            n845 = call "sumofphotons.vi"("s"=FALSE) -> ("sum of photons out"=w895:u32[][][][])  [unwired: 1 in]
                            n846 = property on="router" class="Ring (strict)"() -> ("Value"=w900:u8)  [unwired: 2 in, 2 out]
                            n847 = property on="plane" class="DigNum (strict)"() -> ("Value"=w899:u32)  [unwired: 2 in, 2 out]
                            n848 = property on="threshold" class="Clust (strict)"() -> ("Value"=w894:cluster{"max":u32, "min":u32})  [unwired: 2 in, 2 out]
                            n849 = property on="RGB or false color?" class="Bool (strict)"() -> ("Value"=w898:bool)  [unwired: 2 in, 2 out]
                            n850 = call "OnlinePic.vi"("action"=T2."ini" ("Enum"), "RGB/False"=w898, "Threshold (max)"=w894, "plane"=w899, "router channel"=w900, "Array"=w895) -> ()  [unwired: 1 in, 5 out]
                          }
                          frame #6 {
                            n851 = call "ViewImageSetnew.vi"("action"=enum16{"Display", "change", "Get", "Set"}."Get" ("Enum")) -> ("Image Settings"=w906:T11)  [unwired: 2 in]
                            n852 = Unbundle By Name(w906) -> ("Image Size (pixel).z"=w905:u32)
                            n853 = case shown="0" w905 {
                              tunnel: [i8 2 w910] -> w904
                              tunnel: [u8 0 w910] -> w903
                              frame #0 {
                              }
                              frame #1 {
                                w910 = u8 0
                              }
                            }
                            n854 = property on="plane" class="DigNum (strict)"("Disabled"=w904, "Value"=w903) -> ()  [unwired: 2 in, 2 out]
                          }
                          frame #7 {
                            w911 = u8 0
                            n855 = property on="Image LOADED" class="Boolean (strict)"("Blinking"=FALSE, "Value"=TRUE ("Image LOADED")) -> ()  [unwired: 2 in, 2 out]
                            n856 = property on="Lifetime pick" class="Boolean"("Disabled"=w911) -> ()  [unwired: 2 in, 2 out]
                            n857 = property on="RGB or false color?" class="Boolean (strict)"("Disabled"=w911) -> ()  [unwired: 2 in, 2 out]
                            n858 = property on="router" class="Ring (strict)"("Disabled"=w911) -> ()  [unwired: 2 in, 2 out]
                            n859 = property on="16bit" class="Boolean"("Disabled"=w911) -> ()  [unwired: 2 in, 2 out]
                            n860 = property on="threshold" class="Clust (strict)"("Disabled"=w911) -> ()  [unwired: 2 in, 2 out]
                            n861 = property on="coincidence spot" class="Boolean"("Disabled"=w911) -> ()  [unwired: 2 in, 2 out]
                            n862 = property on="TAC Window" class="Boolean"("Disabled"=w911) -> ()  [unwired: 2 in, 2 out]
                            n863 = property on="Export" class="Bool"("Disabled"=w911) -> ()  [unwired: 2 in, 2 out]
                            n864 = property on="coincidence\nimage" class="Bool"("Disabled"=w911) -> ()  [unwired: 2 in, 2 out]
                          }
                          frame #8 {
                            n865 = property on="Ampel" class="Clust (strict)"("Value"=cluster{"RED":bool, "RED 2":bool, "RED 3":bool} {"RED"=FALSE, "RED 2"=FALSE, "RED 3"=TRUE} ("Ampel")) -> ()  [unwired: 2 in, 2 out]
                          }
                          frame #9 {
                            n866 = property on="LOADED HDR" class="Boolean (strict)"() -> ("Value"=w916:bool)  [unwired: 2 in, 2 out]
                            n867 = case shown="True" w916 {
                              frame #0 {
                              }
                              frame #1 {
                                w918 = FALSE ("Boolean")
                                w917 = u8 2 ("Disabled")
                                n868 = property on="Image LOADED" class="Boolean (strict)"("Value"=w918, "Blinking"=w918) -> ()  [unwired: 2 in, 2 out]
                                n869 = property on="Spotfinder" class="Boolean"("Disabled"=w917) -> ()  [unwired: 2 in, 2 out]
                                n870 = property on="TAC Window" class="Boolean"("Disabled"=w917) -> ()  [unwired: 2 in, 2 out]
                                n871 = property on="Export" class="Boolean"("Disabled"=w917) -> ()  [unwired: 2 in, 2 out]
                                n872 = property on="View Image Settings" class="Boolean"("Disabled"=w917) -> ()  [unwired: 2 in, 2 out]
                                n873 = property on="View FIFO Settings" class="Boolean"("Disabled"=w917) -> ()  [unwired: 2 in, 2 out]
                              }
                            }
                          }
                          frame #10 {
                            n874 = stacked-sequence {
                              frame #0 {
                                n875 = call "TempRefnum.vi"("change?"=FALSE) -> ("refnum out"=w921:refnum<k1>)  [unwired: 1 in]
                                n876 = Close File(refnum=w921) -> (error out=w919:errorcluster)  [unwired: 1 in, 1 out]
                                n877 = call "HandleError.vi"("error in (no error)"=w919) -> ()
                              }
                              frame #1 {
                                n878 = call "TotalRecall_Reload.vi"() -> ("gap"=w922:i32, "invalid"=w923:i32, "valid"=w924:i32)  [unwired: 4 in, 1 out]
                                n879 = property on="total" class="DigNum (strict)"("Value"=w924) -> ()  [unwired: 2 in, 2 out]
                                n880 = property on="invalid" class="DigNum (strict)"("Value"=w923) -> ()  [unwired: 2 in, 2 out]
                                n881 = property on="gap" class="DigNum (strict)"("Value"=w922) -> ()  [unwired: 2 in, 2 out]
                              }
                            }
                          }
                        }
                      }
                    }
                    frame #1 {
                      n882 = control-ref of="notes"() -> (w925:refnum<vi>)
                      n883 = stacked-sequence {
                        tunnel: w925 -> [w930 w937 _]
                        frame #0 {
                          n884 = property class="Str"(reference=w930) -> (reference out=w929:refnum<vi>, "Value"=w928:string)  [unwired: 1 in, 1 out]
                          n885 = property on="Ampel" class="Clust (strict)"("Value"=cluster{"RED":bool, "YELLOW":bool, "GREEN":bool} {"RED"=FALSE, "YELLOW"=FALSE, "GREEN"=FALSE} ("Ampel")) -> ("Controls[]"=w934:refnum<vi>[])  [unwired: 2 in, 2 out]
                          n886 = Concatenate Strings(w928, "\n- spotfinder\n") -> (w927:string)
                          n887 = Index Array(array=w934, index=1) -> (element=w932:refnum<vi>)
                          n888 = property class="Ctl"(reference=w932, "Blinking"=TRUE) -> ()  [unwired: 1 in, 2 out]
                          n889 = property class="Str"(reference=w929, "Value"=w927) -> ()  [unwired: 1 in, 2 out]
                        }
                        frame #1 {
                          n890 = control-ref of="plane"() -> (w939:refnum<vi>)
                          n891 = control-ref of="TACwinLoaded?"() -> (w941:refnum<vi>)
                          n892 = control-ref of="16btimage?"() -> (w940:refnum<vi>)
                          n893 = control-ref of="router"() -> (w938:refnum<vi>)
                          n894 = control-ref of="Image Path"() -> (w942:refnum<vi>)
                          n895 = control-ref of="Int duplex?"() -> (w943:refnum<vi>)
                          n896 = call "SpotFinder.vi"("first scan?"=TRUE, "Int duplex?"=w943, "notes"=w937, "router 3"=w938, "plane 2"=w939, "Image Path"=w942, "16bit?"=w940, "TACwinLoaded?"=w941) -> ()  [unwired: 3 in]
                        }
                        frame #2 {
                          n897 = property on="Ampel" class="Clust (strict)"("Value"=cluster{"RED":bool, "YELLOW":bool, "GREEN":bool} {"RED"=FALSE, "YELLOW"=FALSE, "GREEN"=TRUE} ("Ampel")) -> ("Controls[]"=w947:refnum<vi>[])  [unwired: 2 in, 2 out]
                          n898 = Index Array(array=w947, index=1) -> (element=w945:refnum<vi>)
                          n899 = property class="Ctl"(reference=w945, "Blinking"=FALSE) -> ()  [unwired: 1 in, 2 out]
                        }
                      }
                    }
                  }
                }
              }
              frame #14 {
                n900 = call "spotfindsettings.vi"("Enum"=T1."load") -> ()  [unwired: 8 in, 3 out]
                n901 = call "StandardSettings.vi"("Enum"=enum16{"Load", "get", "Save", "set"}."Load") -> ("StandardSettings"=w954:T9)  [unwired: 4 in]
                n902 = Unbundle By Name(w954) -> ("threshold"=w950:cluster{"max":u32, "min":u32}, "RGB or false color"=w955:bool)
                n903 = property on="Image LOADED" class="Bool (strict)"() -> ("Value"=w953:bool)  [unwired: 2 in, 2 out]
                n904 = Select(t=u8 0 ("Disabled"), s=w953, f=u8 2) -> (s? t:f=w949:u8)
                n905 = property on="RGB or false color?" class="Boolean (strict)"("Disabled"=w949, "Value"=w955) -> ()  [unwired: 2 in, 2 out]
                n906 = property on="threshold" class="Clust (strict)"("Disabled"=w949, "Value"=w950) -> ()  [unwired: 2 in, 2 out]
              }
              frame #15 {
                n907 = stacked-sequence {
                  frame #0 {
                    n908 = call "StandardSettings.vi"("Enum"=enum16{"Load", "get", "Save", "set"}."Save") -> ()  [unwired: 4 in, 1 out]
                  }
                  frame #1 {
                    n909 = call "spotfindsettings.vi"("Enum"=T1."save") -> ()  [unwired: 8 in, 3 out]
                  }
                }
              }
              frame #16 {
                n910 = control-ref of="notes"() -> (w960:refnum<vi>)
                n911 = call "spotfindsettings.vi"("Enum"=enum16{"Display", "change", "get"}."Display", "notes 2"=w960) -> ()  [unwired: 7 in, 3 out]
              }
              frame #17 {
                n912 = property on="Image Path" class="Path"() -> ("Value"=w962:path)  [unwired: 2 in, 2 out]
                n913 = Not A Number/Path/Refnum?(number/path/refnum=w962) -> (NaN/Path/Refnum?=w963:bool)
                n914 = case shown="False" w963 {
                  tunnel: w962 -> [w971 _]
                  frame #0 {
                    n915 = call "scanSubDir.vi"("path"=w971) -> ("Array"=w969:path[])
                    n916 = call "ScanSubDirGlobal.vi"("set"=TRUE, "Array 2"=w969) -> ()  [unwired: 1 out]
                    n917 = Path To String(path=w969) -> (string=w968:string[])
                    n918 = Array Size(array=w968) -> (size(s)=w967:i32)
                    n919 = Not Equal To 0?(x=w967) -> (x != 0?=w966:bool)
                    n920 = Not(x=w966) -> (.not. x?=w965:bool)
                    n921 = property on="Header Path Ring" class="Ring (strict)"("Strings []"=w968, "Visible"=w966, "Disabled"=u8 0) -> ()  [unwired: 2 in, 2 out]
                    n922 = property on="Image Path" class="Path"("Visible"=w965) -> ()  [unwired: 2 in, 2 out]
                  }
                  frame #1 {
                    n923 = property on="Image Path" class="Path"("Visible"=TRUE) -> ()  [unwired: 2 in, 2 out]
                    n924 = property on="Header Path Ring" class="Ring (strict)"("Visible"=FALSE) -> ()  [unwired: 2 in, 2 out]
                  }
                }
              }
              frame #18 {
                n925 = property on="plane" class="DigNum (strict)"() -> ("Disabled"=w975:u8)  [unwired: 2 in, 2 out]
                n926 = Not Equal To 0?(x=w975) -> (x != 0?=w974:bool)
                n927 = case shown="False" w974 {
                  frame #0 {
                    n928 = call "3dview.vi"() -> ()  [unwired: 7 in]
                  }
                  frame #1 {
                  }
                }
              }
              frame #19 {
                n929 = call "ProfileXY.vi"() -> ()  [unwired: 1 in]
              }
              frame #20 {
                n930 = property on="Image LOADED" class="Boolean (strict)"() -> ("Value"=w976:bool)  [unwired: 2 in, 2 out]
                n931 = case shown="True" w976 {
                  frame #0 {
                  }
                  frame #1 {
                    n932 = call "ConcidenceTesting.vi"() -> ()  [unwired: 1 in]
                  }
                }
              }
            }
          }
          event #18 {
            n933 = event-data() -> ()  [unwired: 1 in, 5 out]
            n934 = property on="LOADED HDR" class="Bool (strict)"() -> ("Value"=w978:bool)  [unwired: 2 in, 2 out]
            n935 = case shown="True" w978 {
              frame #0 {
                n936 = One Button Dialog(message="No data loaded.") -> ()  [unwired: 1 in, 1 out]
              }
              frame #1 {
                n937 = stacked-sequence {
                  frame #0 {
                    n938 = property on="Ampel" class="Clust (strict)"("Value"=cluster{"RED":bool, "RED 2":bool, "RED 3":bool} {"RED"=FALSE, "RED 2"=FALSE, "RED 3"=FALSE} ("Ampel")) -> ()  [unwired: 2 in, 2 out]
                    n939 = property on="YELLOW" class="Boolean (strict)"("Blinking"=TRUE) -> ()  [unwired: 2 in, 2 out]
                  }
                  frame #1 {
                    n940 = case shown="True" "View FIFO Settings" {
                      frame #0 {
                      }
                      frame #1 {
                        n941 = call "ViewFIFOSet.vi"("Enum"=enum16{"Display", "change", "Get", "Set"}."Display") -> ()  [unwired: 1 in, 1 out]
                      }
                    }
                    n942 = case shown="True" "View Image Settings" {
                      frame #0 {
                      }
                      frame #1 {
                        n943 = call "ViewImageSetnew.vi"("action"=enum16{"Display", "change", "Get", "Set"}."Display" ("Enum")) -> ()  [unwired: 2 in, 1 out]
                      }
                    }
                  }
                  frame #2 {
                    n944 = property on="Ampel" class="Clust (strict)"("Value"=cluster{"RED":bool, "RED 2":bool, "RED 3":bool} {"RED"=FALSE, "RED 2"=FALSE, "RED 3"=TRUE} ("Ampel")) -> ()  [unwired: 2 in, 2 out]
                    n945 = property on="YELLOW" class="Boolean (strict)"("Blinking"=FALSE) -> ()  [unwired: 2 in, 2 out]
                  }
                }
              }
            }
          }
          event #19 {
            n946 = event-data() -> ()  [unwired: 1 in, 1 out]
          }
          event #20 {
            n947 = event-data() -> ()  [unwired: 1 in, 3 out]
            n948 = Two Button Dialog(message="Do you really want to quit ANNA_linescan?") -> (T button?=w991:bool)  [unwired: 2 in]
            n949 = Not(x=w991) -> (.not. x?=w990:bool)
            n950 = event-data("Discard?"=w990) -> ()  [unwired: 1 in, 1 out]
          }
        }
      }
    }
    frame #5 {
      n951 = Path To String(path=path "") -> (string=w995:string)
      n952 = Concatenate Strings("Anna_linescan " ("string"), w995) -> (w997:string)
      n953 = call "sumofphotons.vi"("s"=TRUE, "sum of photons"=u32[][][][] []) -> ()  [unwired: 1 out]
      n954 = property class="VI"("Front Panel Window:Title"=w997) -> ()  [unwired: 2 in, 2 out]
      n955 = call "IMAQ GetPalette"() -> ()  [unwired: 5 in, 2 out]
      n956 = call "IMAQ WindClose"("Close All Windows (False)"=TRUE ("Close All Windows (N)")) -> ("error out"=w1001:errorcluster)  [unwired: 5 in]
      n957 = property class="VI"("Front Panel Window:Open"=TRUE) -> ()  [unwired: 2 in, 2 out]
      n958 = call "IMAQ WindToolsClose"("error in (no error)"=w1001) -> ()  [unwired: 5 in, 1 out]
      n959 = property on="Ampel" class="Clust (strict)"("Value"=cluster{"RED":bool, "RED 2":bool, "RED 3":bool} {"RED"=FALSE, "RED 2"=FALSE, "RED 3"=FALSE} ("Ampel")) -> ()  [unwired: 2 in, 2 out]
      n960 = stacked-sequence {
        frame #0 {
          n961 = property on="LOADED HDR" class="Bool (strict)"() -> ("Value"=w1003:bool)  [unwired: 2 in, 2 out]
          n962 = case shown="True" w1003 {
            frame #0 {
            }
            frame #1 {
              n963 = control-ref of="notes"() -> (w1005:refnum<vi>)
              n964 = call "SaveNotes.vi"("Enum"=enum16{"Get Path", "Read", "Save"}."Save", "String"=w1005) -> ()  [unwired: 3 in]
            }
          }
        }
        frame #1 {
          n965 = property on="notes" class="String"("Value"="") -> ()  [unwired: 2 in, 2 out]
        }
      }
      n966 = property on="YELLOW" class="Boolean (strict)"("Blinking"=TRUE) -> ()  [unwired: 2 in, 2 out]
    }
  }
